vi "HYSTERISIS_TEMPERATURE CONTROL.vi"() -> ()   [LabVIEW 2010]
uses:
  <instrlib>/Keithley 24XX/Public/Data/Read (Multiple Points).vi
  <vilib>/Utility/file.llb/Write To Spreadsheet File (DBL).vi
  C/Program Files/National Instruments/LabVIEW 2016/instr.lib/Stanford Research 830/Stanford Research 830.lvlib
  C/Program Files/National Instruments/LabVIEW 2016/instr.lib/Keithley 2450/Keithley 2450.lvlib
  <instrlib>/Keithley 24XX/Keithley 24XX.lvlib
  <vilib>/Analysis/NI_AALBase.lvlib
  C/Program Files/National Instruments/LabVIEW 2016/instr.lib/Lake Shore Cryotronics 331/Lake Shore Cryotronics 331.lvlib
panel:
  out "Kelvin Reading 3":dbl min=0.0 max=1645.0 step=1e-05 format="%^.5e"
  in  "Input (0: A) 3":u16(ring) items=["A", "B"]
  out "TEMPERATURE SET":i32
  out "Loop 1\nHeater Output 2":dbl(slide) min=0.0 max=100.0 step=0.01 scale=0.0..100.0 scale format="%.1f"
  in  "Input (0: A) 2":u16(ring) items=["A", "B"]
  out "Kelvin Reading 2":dbl min=0.0 max=1645.0 step=1e-05 format="%^.5e"
  in  "TEMPERATURE STABLE TIME":i32=1000
  in  "TEMPERATURE POINT":i32
  in  "TEMPERATURE SPACE":i32
  in  "INITIAL temperature":i32
  in  "Loop (0: 1)":u16(ring) items=["1", "2"]
  in  "LAKESHORE":refnum<visa-resource-name>="GPIB0::12::INSTR"
  in  "Gain (P) (0.0)":dbl min=0.0 max=1000.0 step=0.1 format="%.1f"
  in  "Reset (I) (0.0)":dbl min=0.0 max=1000.0 step=0.1 format="%.1f"
  in  "Manual Output (0.000)":dbl min=0.0 max=100.0 step=0.001 format="%.3f"
  in  "Heater Range (0: Off)":u16(ring) items=["Off", "Low (0.5W)", "Med (5W)", "High (50W)"]
  in  "Rate (D) (0)":dbl min=0.0 max=200.0 step=1.0
  in  "Configure (False)":bool
  in  "Parameter2 (1: X)  2":u16(ring)=4 items=["X"=1, "Y"=2, "R"=3, "Theta"=4, "Channel 1"=5, "Channel 2"=6, "Aux In 1"=7, "Aux In 2"=8, "Aux In 3"=9, "Aux In 4"=10]
  out "PHASE":dbl=180.0
  out "LOCKIN2\n-THETA":cluster{dbl[], dbl[]}(graph)={[0.0, 0.0, 0.0, 0.0, 0.0, 0.0, 2.3842e-07, 0.0, 0.0, 0.0, 0.0, 0.0, 0.0, 0.0, 0.0, 0.0, 0.0, 0.0, 0.0, 0.0, 0.0, 0.0, 2.3842e-07, 2.3842e-07, 4.76841e-07, 2.3842e-07, 2.3842e-07, 0.0, 0.0, 0.0, 0.0, 0.0, 0.0, 0.0, 0.0, 0.0, 0.0, 2.3842e-07, 2.3842e-07, 2.3842e-07, 0.0, 2.3842e-07, 2.3842e-07, 0.0, 0.0, 0.0, 0.0, 0.0, 0.0, 0.0, 0.0, 0.0, 0.0, 0.0, 2.3842e-07, 2.3842e-07, 2.3842e-07, 2.3842e-07, 0.0, 0.0, 0.0, 0.0, 0.0, 0.0, 0.0, 0.0, 0.0, 0.0, 0.0, 0.0, 0.0, 0.0, 0.0, 0.0, 0.0, 0.0, 0.0, 0.0, 0.0, 0.0, 0.0, 0.0, 0.0, 0.0, 0.0, 0.0, 0.0, 0.0, 0.0, 0.0, 0.0, 0.0, 0.0, 0.0, 0.0, 0.0, 0.0, 0.0, 0.0, 0.0, 0.0, 0.0, 0.0, 0.0, 0.0, 2.3842e-07, 2.3842e-07, 2.3842e-07, 0.0, 0.0, 0.0, 0.0, 0.0, 0.0, 0.0, 0.0, 0.0, 0.0, 0.0, 2.3842e-07, 2.3842e-07, 2.3842e-07, 2.3842e-07, 2.3842e-07, 0.0, 2.3842e-07, 2.3842e-07, 2.3842e-07, 2.3842e-07, 0.0, 0.0, 0.0, 0.0, 0.0, 0.0, 0.0, 0.0, 0.0, 0.0, 0.0, 0.0, 0.0, 0.0, 0.0, 0.0, 0.0, 0.0, 0.0, 0.0, 0.0, 0.0, 4.76841e-07, 9.53682e-07, 1.66894e-06, 2.62262e-06, 4.29156e-06, 6.43733e-06, 9.77522e-06, 1.33515e-05, 1.59742e-05, 1.57357e-05, 7.86787e-06, 9.53682e-07, 0.0, 0.0, 2.3842e-07, 2.3842e-07, 2.3842e-07, 2.3842e-07, 0.0, 0.0, 0.0, 0.0, 0.0, 0.0, 0.0, 0.0, 0.0, 0.0, 2.3842e-07, 2.3842e-07, 2.3842e-07, 0.0, 0.0, 0.0, 0.0, 0.0, 0.0, 0.0, 0.0, 0.0, 0.0, 0.0, 0.0, 0.0, 0.0, 0.0, 2.3842e-07, 2.3842e-07, 2.3842e-07, 4.76841e-07, 2.3842e-07, 0.0, 0.0, 0.0, 0.0, 0.0, 0.0, 0.0, 0.0, 0.0, 0.0, 0.0, 0.0, 0.0, 0.0, 0.0, 0.0, 0.0, 0.0, 0.0, 0.0, 0.0, 0.0, 0.0, 0.0, 0.0, 0.0, 0.0, 0.0, 0.0, 0.0, 0.0, 0.0, 0.0, 0.0, 0.0, 0.0, 0.0, 0.0, 2.3842e-07, 0.0, 2.3842e-07, 2.3842e-07, 2.3842e-07, 2.3842e-07, 2.3842e-07, 0.0, 0.0, 0.0, 0.0, 0.0, 2.3842e-07, 2.3842e-07, 4.76841e-07, 4.76841e-07, 4.76841e-07, 2.3842e-07, 2.3842e-07, 0.0, 0.0, 0.0, 0.0, 0.0, 0.0, 0.0, 0.0, 2.3842e-07, 2.3842e-07, 2.3842e-07, 2.3842e-07, 2.3842e-07, 2.3842e-07, 2.3842e-07, 2.3842e-07, 2.3842e-07, 2.3842e-07, 2.3842e-07, 2.3842e-07, 2.3842e-07, 2.3842e-07, 2.3842e-07, 2.3842e-07, 0.0, 0.0, 0.0, 0.0, 0.0, 0.0, 2.3842e-07, 2.3842e-07, 2.3842e-07, 2.3842e-07, 2.3842e-07, 2.3842e-07, 2.3842e-07, 0.0], [180.0, 135.0, 90.0, 45.0, 45.0, 45.0, 0.0, 0.0, 0.0, 0.0, 0.0, 45.0, 45.0, 45.0, 45.0, 45.0, 45.0, 45.0, 45.0, 45.0, 90.0, 90.0, 116.562, 116.562, 108.432, 116.562, 116.562, 135.0, 135.0, 0.0, 0.0, 0.0, 45.0, 45.0, 45.0, 45.0, 45.0, 26.562, 26.562, 0.0, -45.0, -45.0, -63.438, -90.0, -45.0, -45.0, 0.0, 0.0, 0.0, 0.0, 0.0, 0.0, 90.0, 45.0, 26.562, 26.562, 26.562, 26.562, 45.0, 90.0, 90.0, 0.0, 0.0, -90.0, -90.0, -90.0, -90.0, 0.0, 0.0, 0.0, 0.0, 0.0, 0.0, 90.0, 90.0, 90.0, 90.0, 180.0, -135.0, -135.0, -135.0, 0.0, 0.0, 0.0, 0.0, -45.0, 0.0, 45.0, 45.0, 45.0, 45.0, 45.0, 45.0, 90.0, 0.0, 0.0, -90.0, -90.0, -90.0, -90.0, 0.0, 0.0, 45.0, 45.0, 45.0, 63.438, 63.438, 90.0, 45.0, 90.0, 90.0, 0.0, 0.0, -45.0, -45.0, -45.0, -45.0, -45.0, -45.0, -63.438, -63.438, -90.0, -90.0, -90.0, -63.438, -26.562, 0.0, 0.0, 26.562, 45.0, 45.0, 0.0, -45.0, -45.0, -90.0, 0.0, 45.0, 45.0, 0.0, 0.0, 0.0, 45.0, 45.0, 45.0, 45.0, 45.0, 90.0, 90.0, 135.0, 135.0, 90.0, 71.568, 59.034, 53.13, 49.764, 49.638, 49.086, 49.188, 49.554, 49.59, 49.968, 50.628, 56.31, 135.0, 135.0, 153.438, 180.0, 180.0, 180.0, 180.0, -135.0, -90.0, -90.0, -45.0, -45.0, -45.0, -45.0, -45.0, -45.0, 0.0, 26.562, 26.562, 45.0, 45.0, 0.0, 0.0, 0.0, 90.0, 90.0, 90.0, 45.0, 45.0, 45.0, 45.0, 0.0, -45.0, -45.0, -63.438, -63.438, -63.438, -45.0, -26.562, -45.0, -45.0, -45.0, -45.0, -90.0, -90.0, 0.0, 0.0, 0.0, 0.0, 0.0, 0.0, 0.0, -45.0, -45.0, -45.0, -90.0, 0.0, 90.0, 90.0, 90.0, 90.0, 45.0, 45.0, 45.0, 45.0, 45.0, 45.0, 0.0, 0.0, 0.0, 0.0, 0.0, -45.0, -45.0, -45.0, -90.0, -90.0, -63.438, -45.0, -26.562, 0.0, 0.0, -26.562, -26.562, -45.0, -45.0, -45.0, -45.0, -45.0, 0.0, 26.562, 18.432, 18.432, 18.432, 26.562, 26.562, 45.0, 45.0, 90.0, 90.0, 0.0, 0.0, -45.0, -45.0, -26.562, -26.562, -26.562, -26.562, 0.0, 0.0, 0.0, 0.0, 0.0, 0.0, 0.0, 0.0, 26.562, 26.562, 26.562, 0.0, 0.0, 0.0, 45.0, 45.0, 0.0, 0.0, 0.0, 0.0, 0.0, 26.562, 26.562, 0.0, 0.0, 0.0]}
  in  "Parameter (1: X) 2":u16(ring)=3 items=["X"=1, "Y"=2, "R"=3, "Theta"=4, "Channel 1"=5, "Channel 2"=6, "Aux In 1"=7, "Aux In 2"=8, "Aux In 3"=9, "Aux In 4"=10]
  out "R Measurement 2":dbl
  out "LOVK2-r":cluster{dbl[], dbl[]}(graph)={[0.0, 0.0, 0.0, 0.0, 0.0, 0.0, 2.3842e-07, 0.0, 0.0, 0.0, 0.0, 0.0, 0.0, 0.0, 0.0, 0.0, 0.0, 0.0, 0.0, 0.0, 0.0, 0.0, 2.3842e-07, 2.3842e-07, 4.76841e-07, 2.3842e-07, 2.3842e-07, 0.0, 0.0, 0.0, 0.0, 0.0, 0.0, 0.0, 0.0, 0.0, 0.0, 2.3842e-07, 2.3842e-07, 2.3842e-07, 0.0, 2.3842e-07, 2.3842e-07, 0.0, 0.0, 0.0, 0.0, 0.0, 0.0, 0.0, 0.0, 0.0, 0.0, 0.0, 2.3842e-07, 2.3842e-07, 2.3842e-07, 2.3842e-07, 0.0, 0.0, 0.0, 0.0, 0.0, 0.0, 0.0, 0.0, 0.0, 0.0, 0.0, 0.0, 0.0, 0.0, 0.0, 0.0, 0.0, 0.0, 0.0, 0.0, 0.0, 0.0, 0.0, 0.0, 0.0, 0.0, 0.0, 0.0, 0.0, 0.0, 0.0, 0.0, 0.0, 0.0, 0.0, 0.0, 0.0, 0.0, 0.0, 0.0, 0.0, 0.0, 0.0, 0.0, 0.0, 0.0, 0.0, 2.3842e-07, 2.3842e-07, 2.3842e-07, 0.0, 0.0, 0.0, 0.0, 0.0, 0.0, 0.0, 0.0, 0.0, 0.0, 0.0, 2.3842e-07, 2.3842e-07, 2.3842e-07, 2.3842e-07, 2.3842e-07, 0.0, 2.3842e-07, 2.3842e-07, 2.3842e-07, 2.3842e-07, 0.0, 0.0, 0.0, 0.0, 0.0, 0.0, 0.0, 0.0, 0.0, 0.0, 0.0, 0.0, 0.0, 0.0, 0.0, 0.0, 0.0, 0.0, 0.0, 0.0, 0.0, 0.0, 4.76841e-07, 9.53682e-07, 1.66894e-06, 2.62262e-06, 4.29156e-06, 6.43733e-06, 9.77522e-06, 1.33515e-05, 1.59742e-05, 1.57357e-05, 7.86787e-06, 9.53682e-07, 0.0, 0.0, 2.3842e-07, 2.3842e-07, 2.3842e-07, 2.3842e-07, 0.0, 0.0, 0.0, 0.0, 0.0, 0.0, 0.0, 0.0, 0.0, 0.0, 2.3842e-07, 2.3842e-07, 2.3842e-07, 0.0, 0.0, 0.0, 0.0, 0.0, 0.0, 0.0, 0.0, 0.0, 0.0, 0.0, 0.0, 0.0, 0.0, 0.0, 2.3842e-07, 2.3842e-07, 2.3842e-07, 4.76841e-07, 2.3842e-07, 0.0, 0.0, 0.0, 0.0, 0.0, 0.0, 0.0, 0.0, 0.0, 0.0, 0.0, 0.0, 0.0, 0.0, 0.0, 0.0, 0.0, 0.0, 0.0, 0.0, 0.0, 0.0, 0.0, 0.0, 0.0, 0.0, 0.0, 0.0, 0.0, 0.0, 0.0, 0.0, 0.0, 0.0, 0.0, 0.0, 0.0, 0.0, 2.3842e-07, 0.0, 2.3842e-07, 2.3842e-07, 2.3842e-07, 2.3842e-07, 2.3842e-07, 0.0, 0.0, 0.0, 0.0, 0.0, 2.3842e-07, 2.3842e-07, 4.76841e-07, 4.76841e-07, 4.76841e-07, 2.3842e-07, 2.3842e-07, 0.0, 0.0, 0.0, 0.0, 0.0, 0.0, 0.0, 0.0, 2.3842e-07, 2.3842e-07, 2.3842e-07, 2.3842e-07, 2.3842e-07, 2.3842e-07, 2.3842e-07, 2.3842e-07, 2.3842e-07, 2.3842e-07, 2.3842e-07, 2.3842e-07, 2.3842e-07, 2.3842e-07, 2.3842e-07, 2.3842e-07, 0.0, 0.0, 0.0, 0.0, 0.0, 0.0, 2.3842e-07, 2.3842e-07, 2.3842e-07, 2.3842e-07, 2.3842e-07, 2.3842e-07, 2.3842e-07, 0.0], [0.0, 0.0, 0.0, 0.0, 0.0, 0.0, 2.3842e-07, 0.0, 0.0, 0.0, 0.0, 0.0, 0.0, 0.0, 0.0, 0.0, 0.0, 0.0, 0.0, 0.0, 0.0, 0.0, 2.3842e-07, 2.3842e-07, 4.76841e-07, 2.3842e-07, 2.3842e-07, 0.0, 0.0, 0.0, 0.0, 0.0, 0.0, 0.0, 0.0, 0.0, 0.0, 2.3842e-07, 2.3842e-07, 2.3842e-07, 0.0, 2.3842e-07, 2.3842e-07, 0.0, 0.0, 0.0, 0.0, 0.0, 0.0, 0.0, 0.0, 0.0, 0.0, 0.0, 2.3842e-07, 2.3842e-07, 2.3842e-07, 2.3842e-07, 0.0, 0.0, 0.0, 0.0, 0.0, 0.0, 0.0, 0.0, 0.0, 0.0, 0.0, 0.0, 0.0, 0.0, 0.0, 0.0, 0.0, 0.0, 0.0, 0.0, 0.0, 0.0, 0.0, 0.0, 0.0, 0.0, 0.0, 0.0, 0.0, 0.0, 0.0, 0.0, 0.0, 0.0, 0.0, 0.0, 0.0, 0.0, 0.0, 0.0, 0.0, 0.0, 0.0, 0.0, 0.0, 0.0, 0.0, 2.3842e-07, 2.3842e-07, 2.3842e-07, 0.0, 0.0, 0.0, 0.0, 0.0, 0.0, 0.0, 0.0, 0.0, 0.0, 0.0, 2.3842e-07, 2.3842e-07, 2.3842e-07, 2.3842e-07, 2.3842e-07, 0.0, 2.3842e-07, 2.3842e-07, 2.3842e-07, 2.3842e-07, 0.0, 0.0, 0.0, 0.0, 0.0, 0.0, 0.0, 0.0, 0.0, 0.0, 0.0, 0.0, 0.0, 0.0, 0.0, 0.0, 0.0, 0.0, 0.0, 0.0, 0.0, 0.0, 4.76841e-07, 9.53682e-07, 1.66894e-06, 2.62262e-06, 4.29156e-06, 6.43733e-06, 9.77522e-06, 1.33515e-05, 1.59742e-05, 1.57357e-05, 7.86787e-06, 9.53682e-07, 0.0, 0.0, 2.3842e-07, 2.3842e-07, 2.3842e-07, 2.3842e-07, 0.0, 0.0, 0.0, 0.0, 0.0, 0.0, 0.0, 0.0, 0.0, 0.0, 2.3842e-07, 2.3842e-07, 2.3842e-07, 0.0, 0.0, 0.0, 0.0, 0.0, 0.0, 0.0, 0.0, 0.0, 0.0, 0.0, 0.0, 0.0, 0.0, 0.0, 2.3842e-07, 2.3842e-07, 2.3842e-07, 4.76841e-07, 2.3842e-07, 0.0, 0.0, 0.0, 0.0, 0.0, 0.0, 0.0, 0.0, 0.0, 0.0, 0.0, 0.0, 0.0, 0.0, 0.0, 0.0, 0.0, 0.0, 0.0, 0.0, 0.0, 0.0, 0.0, 0.0, 0.0, 0.0, 0.0, 0.0, 0.0, 0.0, 0.0, 0.0, 0.0, 0.0, 0.0, 0.0, 0.0, 0.0, 2.3842e-07, 0.0, 2.3842e-07, 2.3842e-07, 2.3842e-07, 2.3842e-07, 2.3842e-07, 0.0, 0.0, 0.0, 0.0, 0.0, 2.3842e-07, 2.3842e-07, 4.76841e-07, 4.76841e-07, 4.76841e-07, 2.3842e-07, 2.3842e-07, 0.0, 0.0, 0.0, 0.0, 0.0, 0.0, 0.0, 0.0, 2.3842e-07, 2.3842e-07, 2.3842e-07, 2.3842e-07, 2.3842e-07, 2.3842e-07, 2.3842e-07, 2.3842e-07, 2.3842e-07, 2.3842e-07, 2.3842e-07, 2.3842e-07, 2.3842e-07, 2.3842e-07, 2.3842e-07, 2.3842e-07, 0.0, 0.0, 0.0, 0.0, 0.0, 0.0, 2.3842e-07, 2.3842e-07, 2.3842e-07, 2.3842e-07, 2.3842e-07, 2.3842e-07, 2.3842e-07, 0.0]}
  in  "Clear Plot 2":bool
  in  "TRIGGER (1:EXTERNAL)":i32=1
  in  "REFERENCE(0:EXTERNAL)":i32
  in  "auto phase 2":bool=TRUE
  in  "manual phase 2":dbl
  in  "harm#2 2":dbl=1.0
  in  "Sine Output Amplitude (1 V) 3":dbl=0.05
  in  "Input Connection (0: Single-Ended Voltage)  2":u16(ring)=1 items=["Single-Ended Voltage", "Differential Voltage", "1 MOhm Current Gain", "100 MOhm Current Gain"]
  in  "frequency 2":dbl=50.0 format="%#_13g"
  in  "lockin-NL":refnum<visa-resource-name>="GPIB0::10::INSTR"
  out "XY Graph 2":cluster{dbl[], dbl[]}(graph)={[0.0, -0.5, -1.0, -1.5, -2.0, -2.5, -3.0, -3.5, -3.0, -2.5, -2.0, -1.5, -1.0, -0.5, 0.0, 0.5, 1.0, 1.5, 2.0, 2.5, 3.0, 3.5, 3.0, 2.5, 2.0, 1.5, 1.0, 0.5, 0.0, 1.64, 1.66, 1.68, 1.7, 1.72, 1.74, 1.76, 1.78, 1.8, 1.82, 1.8399999999999999, 1.8599999999999999, 1.88, 1.9, 1.92, 1.94, 1.96, 1.98, 2.0, 2.02, 2.04, 2.06, 2.08, 2.0999999999999996, 2.12, 2.1399999999999997, 2.16, 2.1799999999999997, 2.2, 2.2199999999999998, 2.24, 2.26, 2.2800000000000002, 2.3, 2.3200000000000003, 2.34, 2.36, 2.38, 2.4, 2.42, 2.44, 2.46, 2.48, 2.5, 2.52, 2.54, 2.56, 2.58, 2.6, 2.62, 2.64, 2.66, 2.6799999999999997, 2.7, 2.7199999999999998, 2.74, 2.76, 2.7800000000000002, 2.8, 2.82, 2.84, 2.86, 2.88, 2.9, 2.92, 2.94, 2.96, 2.98, 3.0, 3.02, 3.04, 3.06, 3.08, 3.1, 3.12, 3.14, 3.16, 3.18, 3.2, 3.2199999999999998, 3.24, 3.26, 3.28, 3.3, 3.32, 3.34, 3.36, 3.38, 3.4, 3.42, 3.44, 3.46, 3.48, 3.5, 3.48, 3.46, 3.44, 3.42, 3.4, 3.38, 3.36, 3.34, 3.3200000000000003, 3.3000000000000003, 3.2800000000000002, 3.2600000000000002, 3.24, 3.22, 3.2, 3.18, 3.16, 3.14, 3.12, 3.1, 3.08, 3.06, 3.04, 3.02, 3.0, 2.98, 2.96, 2.94, 2.92, 2.9, 2.88, 2.86, 2.84, 2.82, 2.8000000000000003, 2.7800000000000002, 2.7600000000000002, 2.74, 2.72, 2.7, 2.68, 2.66, 2.64, 2.62, 2.6, 2.58, 2.56, 2.54, 2.52, 2.5, 2.48, 2.46, 2.44, 2.42, 2.4, 2.38, 2.36, 2.34, 2.32, 2.3000000000000003, 2.2800000000000002, 2.2600000000000002, 2.24, 2.22, 2.2, 2.18, 2.16, 2.14, 2.12, 2.1, 2.08, 2.06, 2.04, 2.02, 2.0, 1.98, 1.96, 1.94, 1.92, 1.9000000000000001, 1.8800000000000001, 1.86, 1.84, 1.82, 1.8, 1.78, 1.76, 1.74, 1.72, 1.7, 1.68, 1.6600000000000001, 1.6400000000000001, 1.62, 1.6, 1.58, 1.56, 1.54, 1.52, 1.5, 1.48, 1.46, 1.44, 1.42, 1.4000000000000001, 1.3800000000000001, 1.36, 1.34, 1.32, 1.3, 1.28, 1.26, 1.24, 1.22, 1.2, 1.18, 1.16, 1.1400000000000001, 1.12, 1.1, 1.08, 1.06, 1.04, 1.02, 1.0, 0.98, 0.96, 0.9400000000000001, 0.92, 0.9, 0.88, 0.86, 0.84, 0.8200000000000001, 0.8, 0.78, 0.76, 0.74, 0.72, 0.7000000000000001, 0.68, 0.66, 0.64, 0.62, 0.6, 0.58, 0.56, 0.54, 0.52, 0.5, 0.48, 0.46, 0.44, 0.42, 0.4, 0.38, 0.36, 0.34, 0.32, 0.3, 0.28, 0.26, 0.24, 0.22, 0.2, 0.18, 0.16, 0.14, 0.12, 0.1, 0.08, 0.06, 0.04, 0.02, 0.0], [180.0, 180.0, 180.0, -135.0, -90.0, -45.0, -63.438, -45.0, 45.0, 71.568, 71.568, 71.568, 90.0, 135.0, 135.0, 135.0, 180.0, -90.0, -90.0, -135.0, 0.0, 0.0, 0.0, -45.0, -45.0, -90.0, -90.0, 0.0, 90.0, -90.0, -45.0, 0.0, 0.0, -18.432, -18.432, -14.034, 0.0, 26.562, 26.562, 45.0, 33.69, 33.69, 18.432, 18.432, 18.432, 18.432, 0.0, 0.0, 0.0, 0.0, 90.0, 90.0, 90.0, 63.438, 90.0, 63.438, 90.0, 90.0, 180.0, -135.0, -90.0, -90.0, -45.0, -63.438, -90.0, -90.0, -90.0, -90.0, -90.0, -135.0, -116.562, -116.562, -116.562, -135.0, -116.562, -135.0, -135.0, 180.0, 135.0, 45.0, 63.438, 71.568, 63.438, 45.0, 0.0, -45.0, -45.0, -56.31, -45.0, -63.438, -63.438, -45.0, -90.0, -90.0, -90.0, -90.0, -90.0, -135.0, -153.438, -153.438, -135.0, -45.0, -45.0, -45.0, 0.0, 45.0, 45.0, 45.0, 45.0, 0.0, -90.0, -90.0, -90.0, -90.0, -63.438, -63.438, -63.438, -26.562, -18.432, -26.562, -26.562, -26.562, 0.0, 0.0, -18.432, -26.562, -63.438, -63.438, -63.438, -45.0, -45.0, -45.0, -45.0, -45.0, -45.0, -45.0, 0.0, 0.0, 45.0, 0.0, -18.432, -18.432, -33.69, -18.432, 0.0, 45.0, 45.0, 63.438, 63.438, 45.0, 26.562, 26.562, 26.562, 45.0, 26.562, 26.562, 18.432, 26.562, 45.0, 45.0, 45.0, 45.0, 45.0, 45.0, 45.0, 45.0, 63.438, 90.0, 90.0, 90.0, 90.0, 45.0, 90.0, 180.0, -135.0, -135.0, -90.0, -90.0, -90.0, -63.438, -45.0, -45.0, 0.0, 45.0, 45.0, -45.0, -45.0, -90.0, -63.438, -63.438, -45.0, -33.69, -33.69, -56.31, -71.568, -71.568, -71.568, -63.438, -71.568, -90.0, -45.0, 0.0, 45.0, 45.0, 63.438, 63.438, 71.568, 63.438, 63.438, 45.0, 90.0, 135.0, 180.0, 180.0, 153.438, 161.568, 180.0, 180.0, 180.0, 180.0, -90.0, -90.0, 0.0, 90.0, 90.0, 90.0, 0.0, -45.0, -45.0, -63.438, -63.438, -63.438, -71.568, -63.438, -63.438, -45.0, -45.0, -63.438, -45.0, -45.0, 0.0, 0.0, 45.0, 0.0, 0.0, 0.0, 90.0, 90.0, 90.0, 0.0, 0.0, 0.0, 0.0, 0.0, 0.0, 0.0, -26.562, -45.0, -45.0, -90.0, -90.0, 0.0, 45.0, 45.0, 63.438, 63.438, 63.438, 45.0, 63.438, 63.438, 63.438, 45.0, 0.0, -90.0, -90.0, -116.562, -135.0, 180.0, 135.0, 90.0, 45.0, 45.0, 0.0, -45.0, -63.438, -45.0, -71.568, -71.568, -63.438, -90.0, 0.0, 90.0, 63.438, 45.0, 26.562, 26.562, 0.0]}
  out "para2 Measurement":dbl=180.0
  in  "Parameter2 (1: X)":u16(ring)=4 items=["X"=1, "Y"=2, "R"=3, "Theta"=4, "Channel 1"=5, "Channel 2"=6, "Aux In 1"=7, "Aux In 2"=8, "Aux In 3"=9, "Aux In 4"=10]
  in  "auto phase":bool
  in  "manual phase":dbl
  in  "harm#2":dbl=2.0
  out "top gate leaking":dbl=-5.0360913356195525e-11
  out "top gate voltage":dbl=-0.0 format="%#_13g"
  in  "Compliance  Level (1uA)":dbl=2e-08
  in  "Source Mode  (0: Voltage)":u16(ring) items=["Voltage", "Current"]
  in  "top gate thickness":dbl=1.0
  in  "bottom gate thickness":dbl=1.0
  in  "pure field (T)/pure doping (F)":bool=TRUE
  in  "Serial Configuration":T1={"Baud Rate"=9600, "Parity"=0, "Data Bits"=8, "Stop Bits"=10, "Flow Control"=0} {"Flow Control" items=["None", "XON/XOFF", "RTS/CTS", "XON/XOFF & RTS/CTS", "DTR/DSR", "XON/XOFF & DTR/DSR"]; "Stop Bits" items=["1.0"=10, "1.5"=15, "2.0"=20]; "Data Bits" items=["7"=7, "8"=8]; "Parity" items=["None", "Odd", "Even", "Mark", "Space"]; "Baud Rate" items=["300"=300, "600"=600, "1200"=1200, "2400"=2400, "4800"=4800, "9600"=9600, "19200"=19200]}
  in  "top gate address":refnum<visa-resource-name>="GPIB0::25::INSTR"
  out "loop run":i32=1
  in  "loop #":i32=1
  in  "Save data or not":bool
  in  "path (folder + filename)":string="D:\\Kedar\\MoS2\\jw7_DJ_bulk_111213\\VvsHtr\\VvsHtr_300K"
  in  "Clear Plot":bool
  out "XY Graph":cluster{dbl[], dbl[]}(graph)={[0.0, -0.5, -1.0, -1.5, -2.0, -2.5, -3.0, -3.5, -3.0, -2.5, -2.0, -1.5, -1.0, -0.5, 0.0, 0.5, 1.0, 1.5, 2.0, 2.5, 3.0, 3.5, 3.0, 2.5, 2.0, 1.5, 1.0, 0.5, 0.0, 1.64, 1.66, 1.68, 1.7, 1.72, 1.74, 1.76, 1.78, 1.8, 1.82, 1.8399999999999999, 1.8599999999999999, 1.88, 1.9, 1.92, 1.94, 1.96, 1.98, 2.0, 2.02, 2.04, 2.06, 2.08, 2.0999999999999996, 2.12, 2.1399999999999997, 2.16, 2.1799999999999997, 2.2, 2.2199999999999998, 2.24, 2.26, 2.2800000000000002, 2.3, 2.3200000000000003, 2.34, 2.36, 2.38, 2.4, 2.42, 2.44, 2.46, 2.48, 2.5, 2.52, 2.54, 2.56, 2.58, 2.6, 2.62, 2.64, 2.66, 2.6799999999999997, 2.7, 2.7199999999999998, 2.74, 2.76, 2.7800000000000002, 2.8, 2.82, 2.84, 2.86, 2.88, 2.9, 2.92, 2.94, 2.96, 2.98, 3.0, 3.02, 3.04, 3.06, 3.08, 3.1, 3.12, 3.14, 3.16, 3.18, 3.2, 3.2199999999999998, 3.24, 3.26, 3.28, 3.3, 3.32, 3.34, 3.36, 3.38, 3.4, 3.42, 3.44, 3.46, 3.48, 3.5, 3.48, 3.46, 3.44, 3.42, 3.4, 3.38, 3.36, 3.34, 3.3200000000000003, 3.3000000000000003, 3.2800000000000002, 3.2600000000000002, 3.24, 3.22, 3.2, 3.18, 3.16, 3.14, 3.12, 3.1, 3.08, 3.06, 3.04, 3.02, 3.0, 2.98, 2.96, 2.94, 2.92, 2.9, 2.88, 2.86, 2.84, 2.82, 2.8000000000000003, 2.7800000000000002, 2.7600000000000002, 2.74, 2.72, 2.7, 2.68, 2.66, 2.64, 2.62, 2.6, 2.58, 2.56, 2.54, 2.52, 2.5, 2.48, 2.46, 2.44, 2.42, 2.4, 2.38, 2.36, 2.34, 2.32, 2.3000000000000003, 2.2800000000000002, 2.2600000000000002, 2.24, 2.22, 2.2, 2.18, 2.16, 2.14, 2.12, 2.1, 2.08, 2.06, 2.04, 2.02, 2.0, 1.98, 1.96, 1.94, 1.92, 1.9000000000000001, 1.8800000000000001, 1.86, 1.84, 1.82, 1.8, 1.78, 1.76, 1.74, 1.72, 1.7, 1.68, 1.6600000000000001, 1.6400000000000001, 1.62, 1.6, 1.58, 1.56, 1.54, 1.52, 1.5, 1.48, 1.46, 1.44, 1.42, 1.4000000000000001, 1.3800000000000001, 1.36, 1.34, 1.32, 1.3, 1.28, 1.26, 1.24, 1.22, 1.2, 1.18, 1.16, 1.1400000000000001, 1.12, 1.1, 1.08, 1.06, 1.04, 1.02, 1.0, 0.98, 0.96, 0.9400000000000001, 0.92, 0.9, 0.88, 0.86, 0.84, 0.8200000000000001, 0.8, 0.78, 0.76, 0.74, 0.72, 0.7000000000000001, 0.68, 0.66, 0.64, 0.62, 0.6, 0.58, 0.56, 0.54, 0.52, 0.5, 0.48, 0.46, 0.44, 0.42, 0.4, 0.38, 0.36, 0.34, 0.32, 0.3, 0.28, 0.26, 0.24, 0.22, 0.2, 0.18, 0.16, 0.14, 0.12, 0.1, 0.08, 0.06, 0.04, 0.02, 0.0], [0.0, 0.0, 0.0, 0.0, 0.0, 0.0, 1.1921e-07, 0.0, 0.0, 1.1921e-07, 1.1921e-07, 1.1921e-07, 1.1921e-07, 0.0, 0.0, 0.0, 0.0, 0.0, 0.0, 0.0, 0.0, 0.0, 0.0, 0.0, 0.0, 0.0, 0.0, 0.0, 0.0, 0.0, 0.0, 0.0, 0.0, 1.1921e-07, 1.1921e-07, 2.3842e-07, 1.1921e-07, 1.1921e-07, 1.1921e-07, 1.1921e-07, 2.3842e-07, 2.3842e-07, 1.1921e-07, 1.1921e-07, 1.1921e-07, 1.1921e-07, 1.1921e-07, 1.1921e-07, 0.0, 0.0, 0.0, 0.0, 0.0, 1.1921e-07, 1.1921e-07, 1.1921e-07, 0.0, 0.0, 0.0, 0.0, 0.0, 0.0, 1.1921e-07, 1.1921e-07, 1.1921e-07, 1.1921e-07, 0.0, 0.0, 0.0, 0.0, 1.1921e-07, 1.1921e-07, 1.1921e-07, 1.1921e-07, 1.1921e-07, 0.0, 0.0, 0.0, 0.0, 0.0, 1.1921e-07, 1.1921e-07, 1.1921e-07, 0.0, 0.0, 0.0, 1.1921e-07, 1.1921e-07, 1.1921e-07, 1.1921e-07, 1.1921e-07, 0.0, 0.0, 0.0, 0.0, 0.0, 0.0, 0.0, 1.1921e-07, 1.1921e-07, 0.0, 0.0, 0.0, 0.0, 1.1921e-07, 0.0, 0.0, 0.0, 0.0, 0.0, 0.0, 0.0, 0.0, 1.1921e-07, 1.1921e-07, 1.1921e-07, 1.1921e-07, 1.1921e-07, 1.1921e-07, 1.1921e-07, 1.1921e-07, 1.1921e-07, 1.1921e-07, 1.1921e-07, 1.1921e-07, 1.1921e-07, 1.1921e-07, 1.1921e-07, 1.1921e-07, 0.0, 0.0, 0.0, 0.0, 0.0, 0.0, 0.0, 0.0, 0.0, 0.0, 1.1921e-07, 1.1921e-07, 1.1921e-07, 2.3842e-07, 1.1921e-07, 0.0, 0.0, 1.1921e-07, 1.1921e-07, 1.1921e-07, 0.0, 1.1921e-07, 1.1921e-07, 1.1921e-07, 0.0, 1.1921e-07, 1.1921e-07, 1.1921e-07, 1.1921e-07, 0.0, 0.0, 0.0, 0.0, 0.0, 0.0, 0.0, 0.0, 1.1921e-07, 1.1921e-07, 0.0, 0.0, 0.0, 0.0, 0.0, 0.0, 0.0, 0.0, 1.1921e-07, 1.1921e-07, 1.1921e-07, 1.1921e-07, 0.0, 0.0, 0.0, 0.0, 0.0, 0.0, 0.0, 1.1921e-07, 1.1921e-07, 1.1921e-07, 1.1921e-07, 2.3842e-07, 2.3842e-07, 2.3842e-07, 1.1921e-07, 1.1921e-07, 1.1921e-07, 1.1921e-07, 1.1921e-07, 1.1921e-07, 0.0, 0.0, 0.0, 0.0, 1.1921e-07, 1.1921e-07, 1.1921e-07, 1.1921e-07, 1.1921e-07, 0.0, 0.0, 0.0, 0.0, 1.1921e-07, 1.1921e-07, 1.1921e-07, 1.1921e-07, 1.1921e-07, 0.0, 0.0, 0.0, 0.0, 0.0, 0.0, 0.0, 0.0, 0.0, 0.0, 0.0, 1.1921e-07, 1.1921e-07, 1.1921e-07, 1.1921e-07, 1.1921e-07, 1.1921e-07, 0.0, 0.0, 1.1921e-07, 0.0, 0.0, 0.0, 0.0, 0.0, 0.0, 0.0, 0.0, 0.0, 0.0, 0.0, 0.0, 0.0, 0.0, 1.1921e-07, 1.1921e-07, 1.1921e-07, 1.1921e-07, 1.1921e-07, 0.0, 0.0, 0.0, 0.0, 0.0, 0.0, 0.0, 1.1921e-07, 1.1921e-07, 0.0, 0.0, 1.1921e-07, 1.1921e-07, 1.1921e-07, 0.0, 0.0, 1.1921e-07, 1.1921e-07, 1.1921e-07, 0.0, 0.0, 0.0, 1.1921e-07, 0.0, 0.0, 0.0, 0.0, 1.1921e-07, 1.1921e-07, 1.1921e-07, 1.1921e-07, 1.1921e-07, 0.0, 0.0, 0.0, 1.1921e-07, 1.1921e-07, 1.1921e-07, 1.1921e-07, 1.1921e-07]}
  out "para1 Measurement":dbl
  in  "Parameter (1: X)":u16(ring)=3 items=["X"=1, "Y"=2, "R"=3, "Theta"=4, "Channel 1"=5, "Channel 2"=6, "Aux In 1"=7, "Aux In 2"=8, "Aux In 3"=9, "Aux In 4"=10]
  out "gate voltage":dbl format="%#_13g"
  out "gate leaking":string="1.034294E-10\n"
  in  "GATE STEP(mv)":i32=500
  in  "GATE Low Value (default 0)":dbl
  in  "GATE High Value":dbl=3.5
  in  "Function (0: Volts) 2":u16(ring) items=["Volts", "Current", "Resistance"]
  in  "Source Compaliance":dbl=1e-08
  in  "back gate address":refnum<visa-resource-name>="GPIB0::18::INSTR"
  in  "SD stabilization(S) 2":dbl=0.1 format="%#_13g"
  in  "Sine Output Amplitude (1 V) 2":dbl=0.2
  in  "LOCKIN-WAIT":dbl=0.1 format="%#_13g"
  in  "frequency":dbl=40.0 format="%#_13g"
  in  "Input Connection (0: Single-Ended Voltage)":u16(ring)=1 items=["Single-Ended Voltage", "Differential Voltage", "1 MOhm Current Gain", "100 MOhm Current Gain"]
  in  "LOCKIN address":refnum<visa-resource-name>="GPIB0::8::INSTR"
  # "Lock-in"
  # "top Gate Setting"
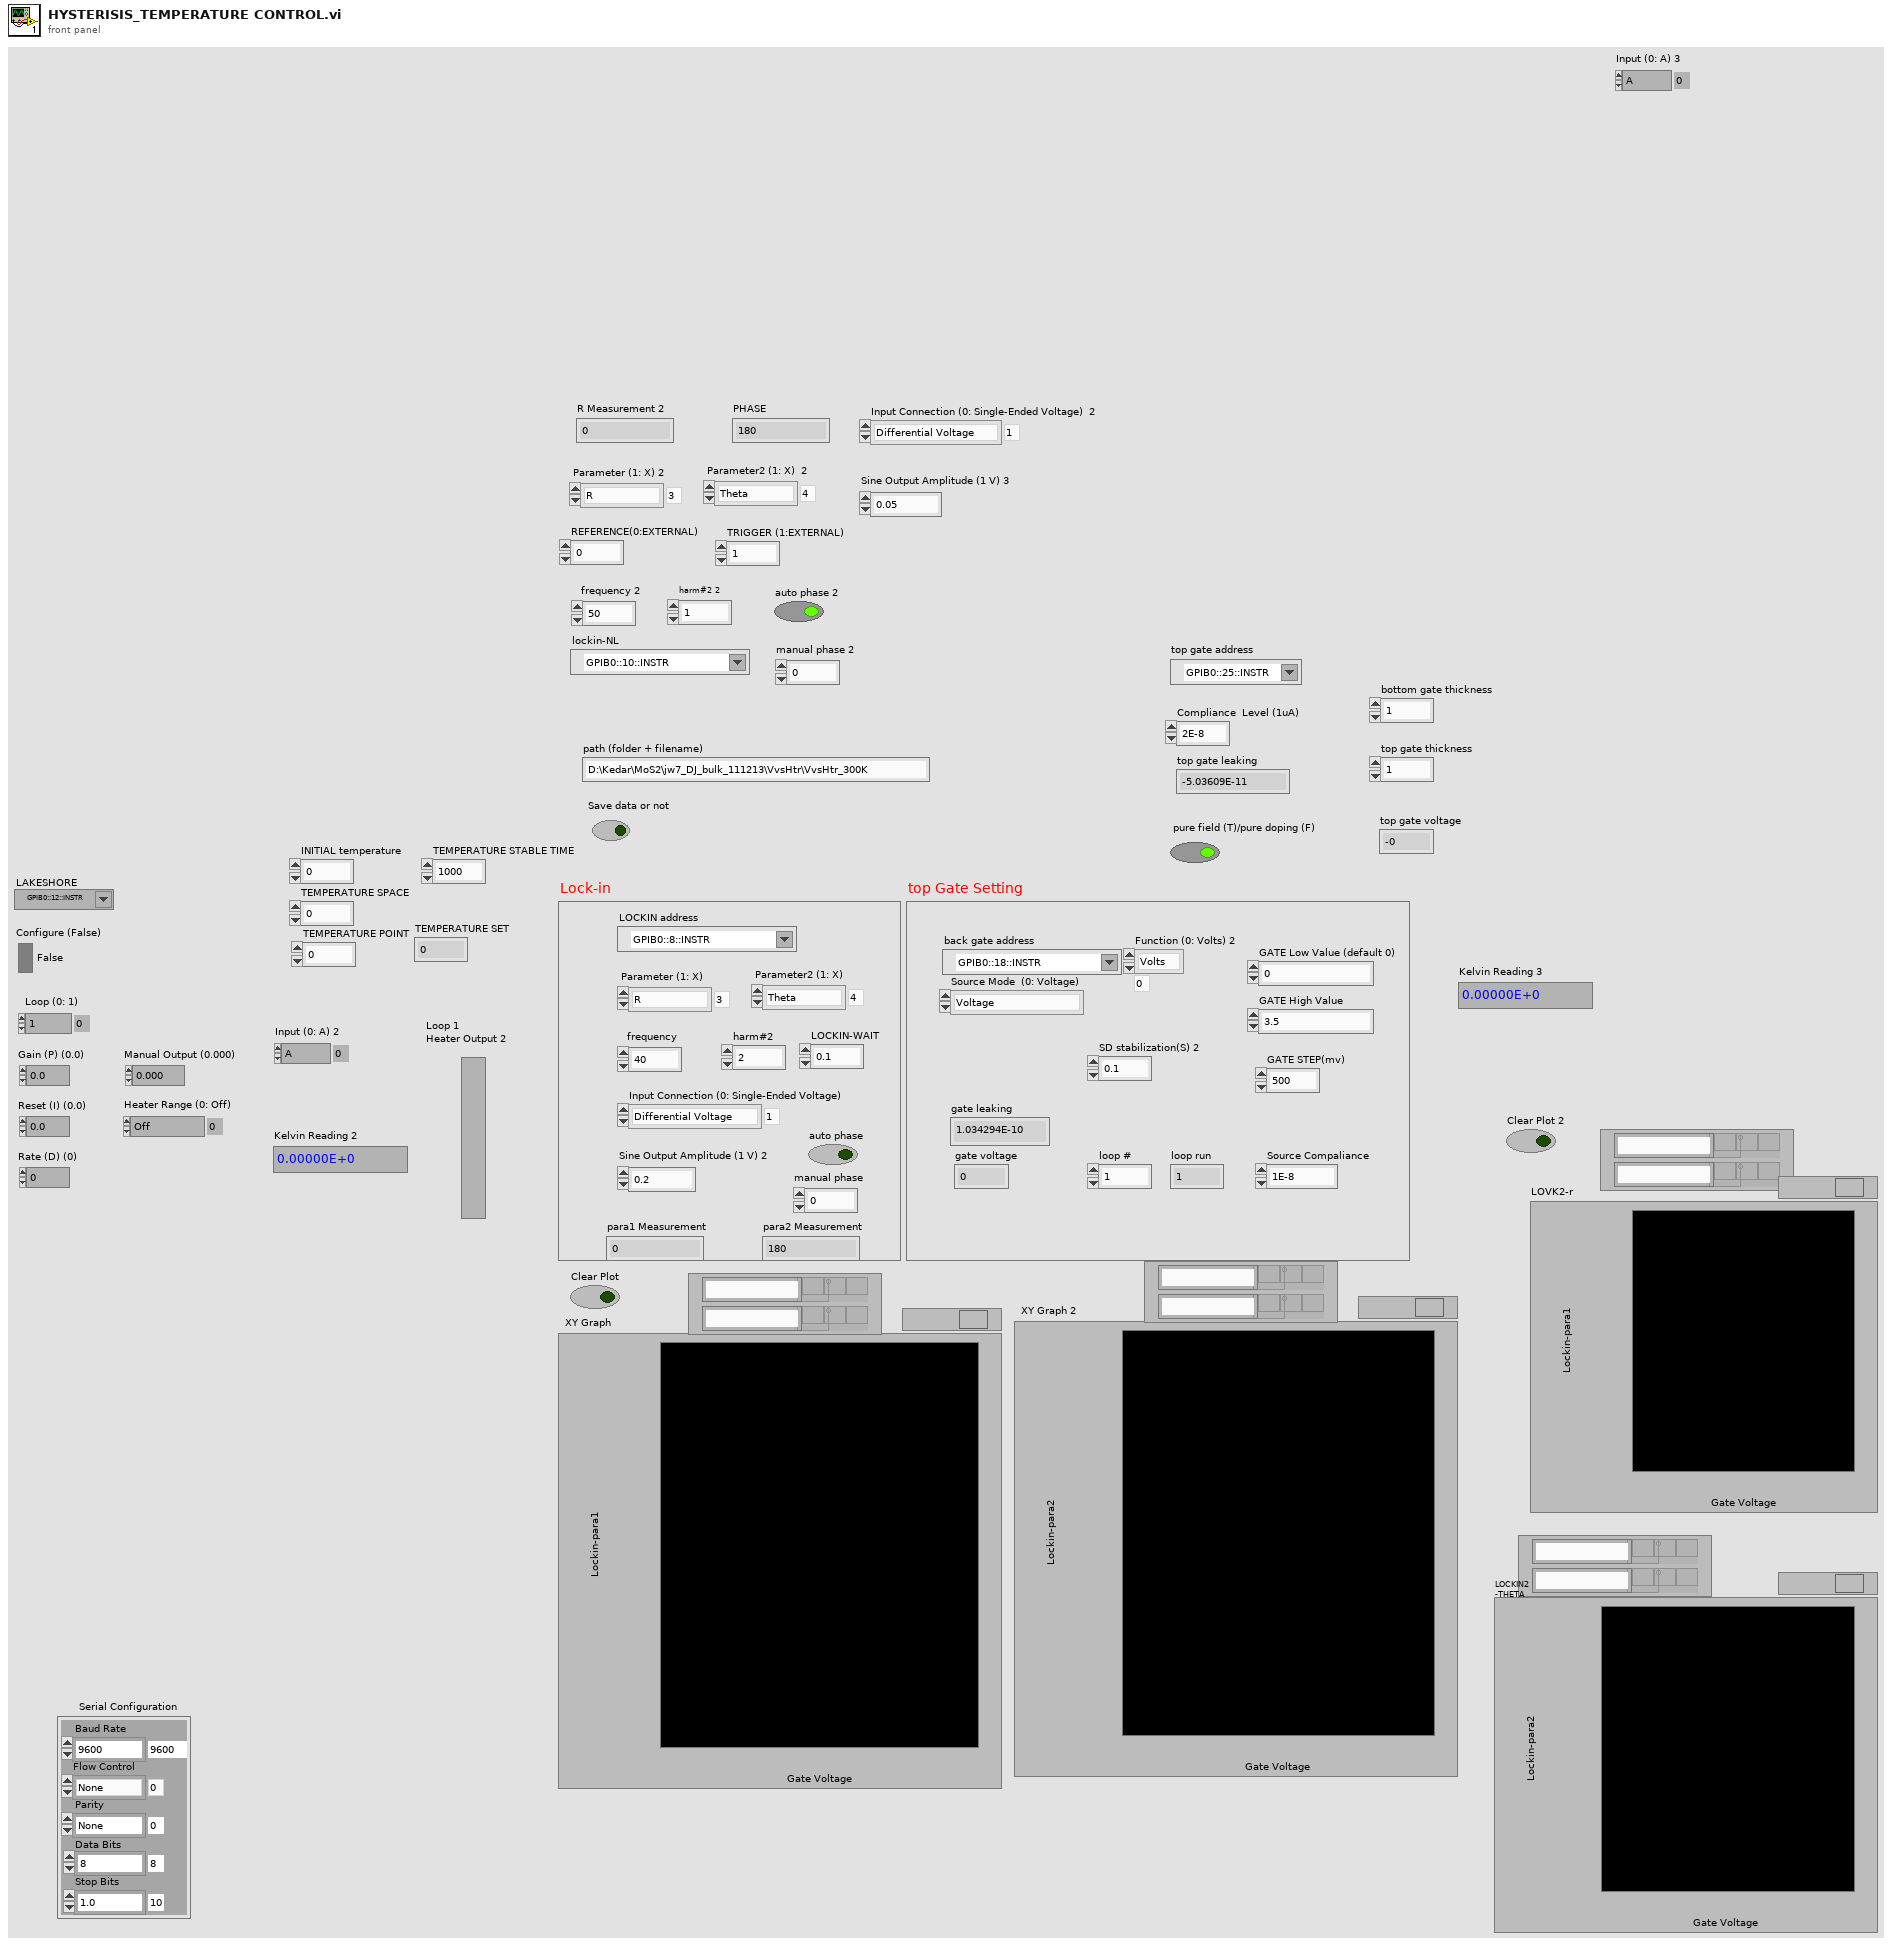
[diagram p1: front panel]
types:
  T1 = cluster{"Baud Rate":u32, "Parity":u16, "Data Bits":u16, "Stop Bits":u16, "Flow Control":u16}
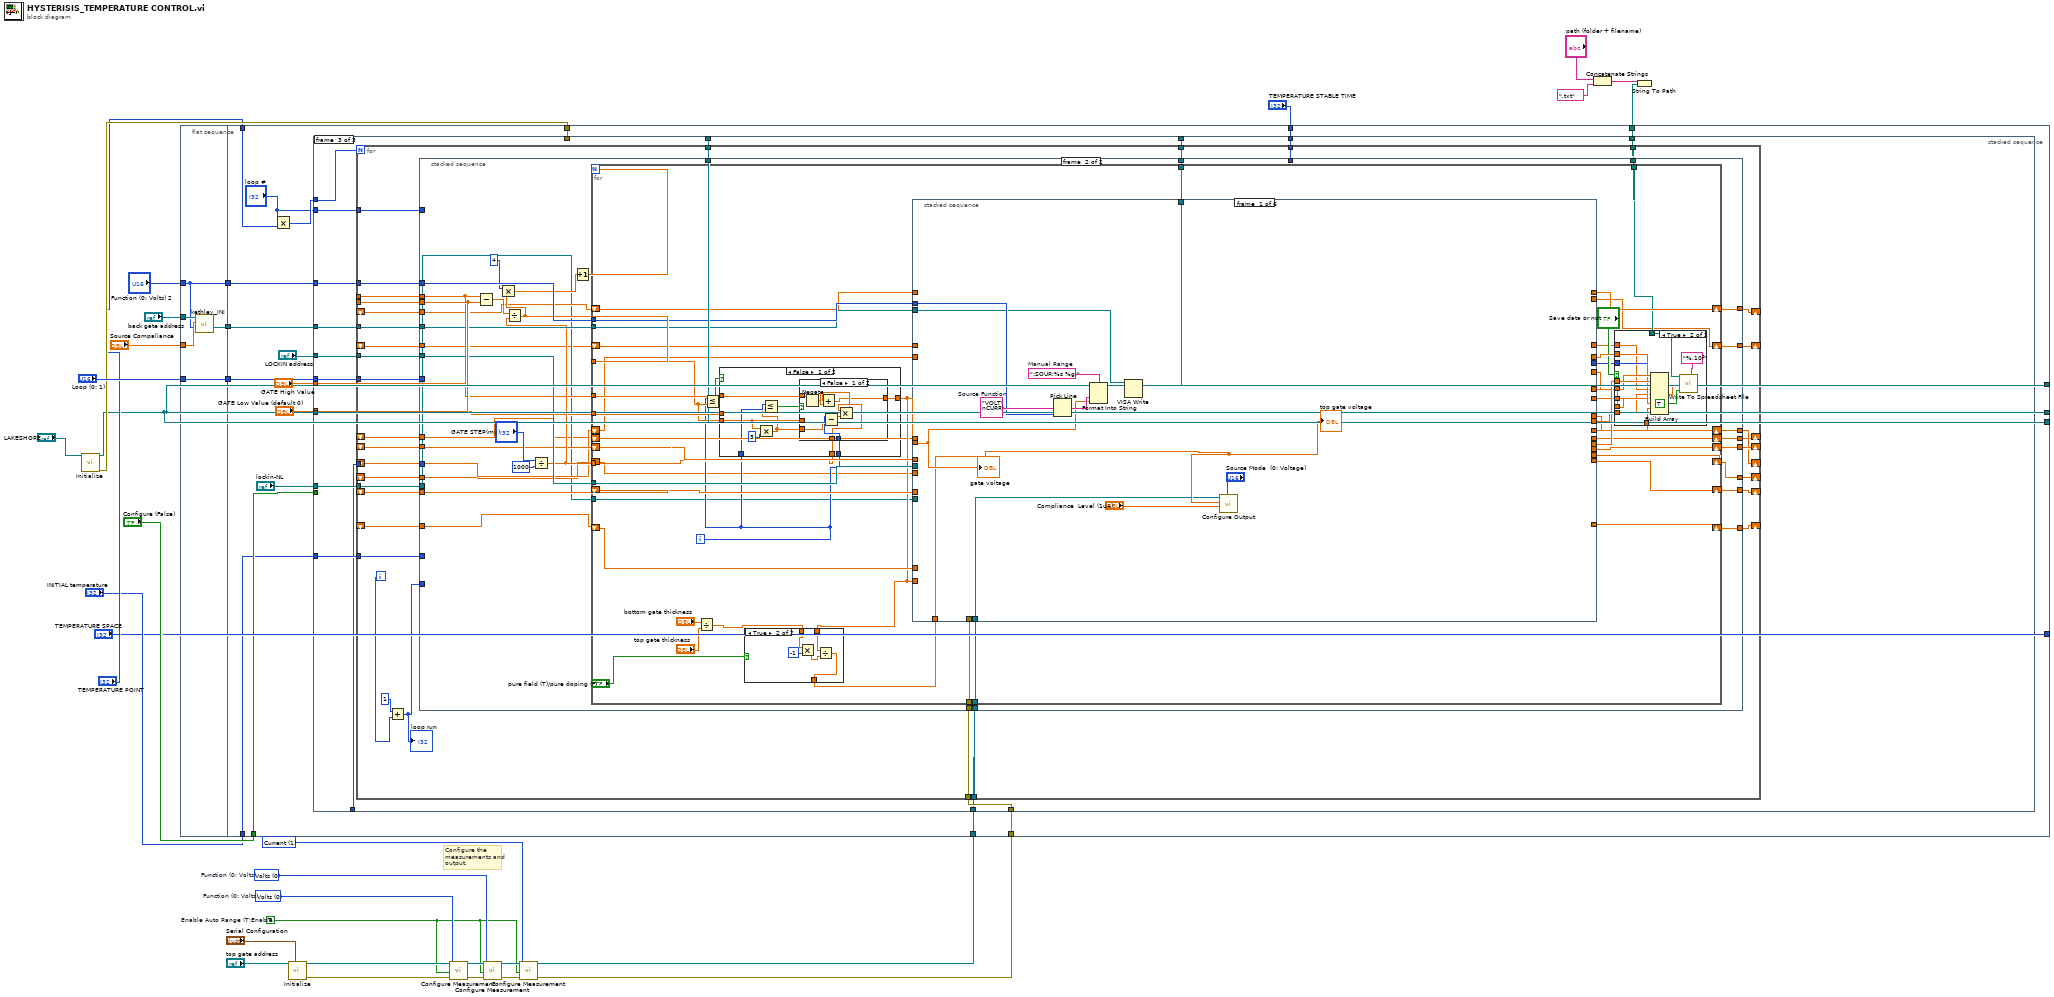
[diagram p0: block diagram]
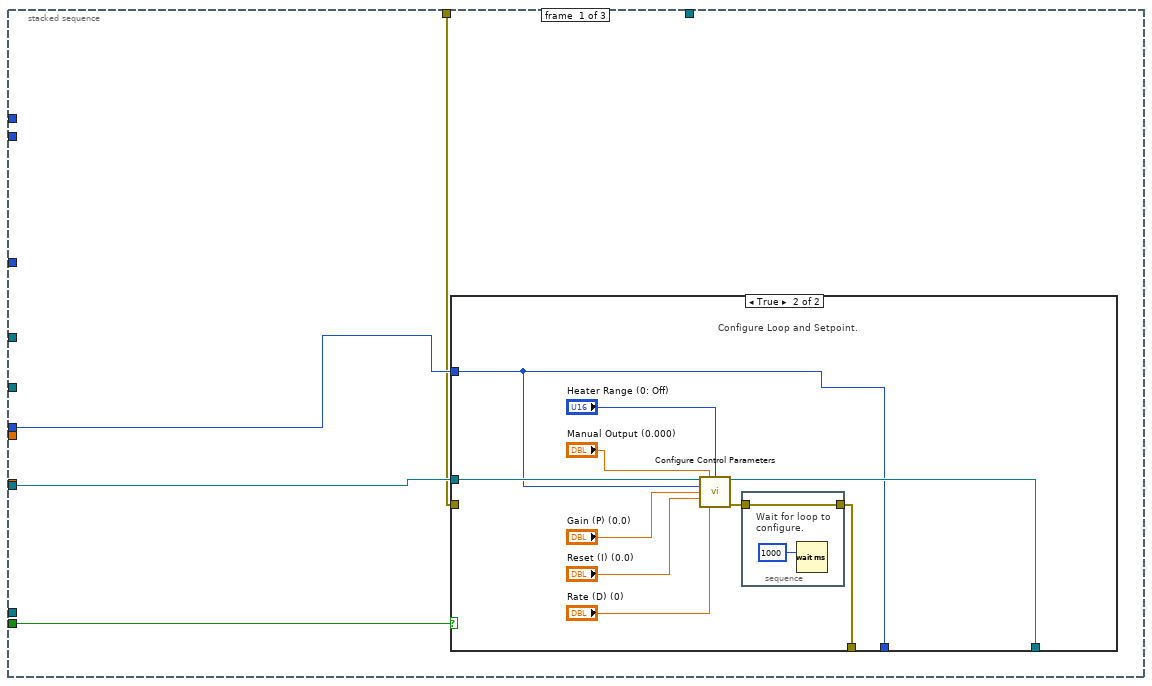
[diagram p2: hidden frame]
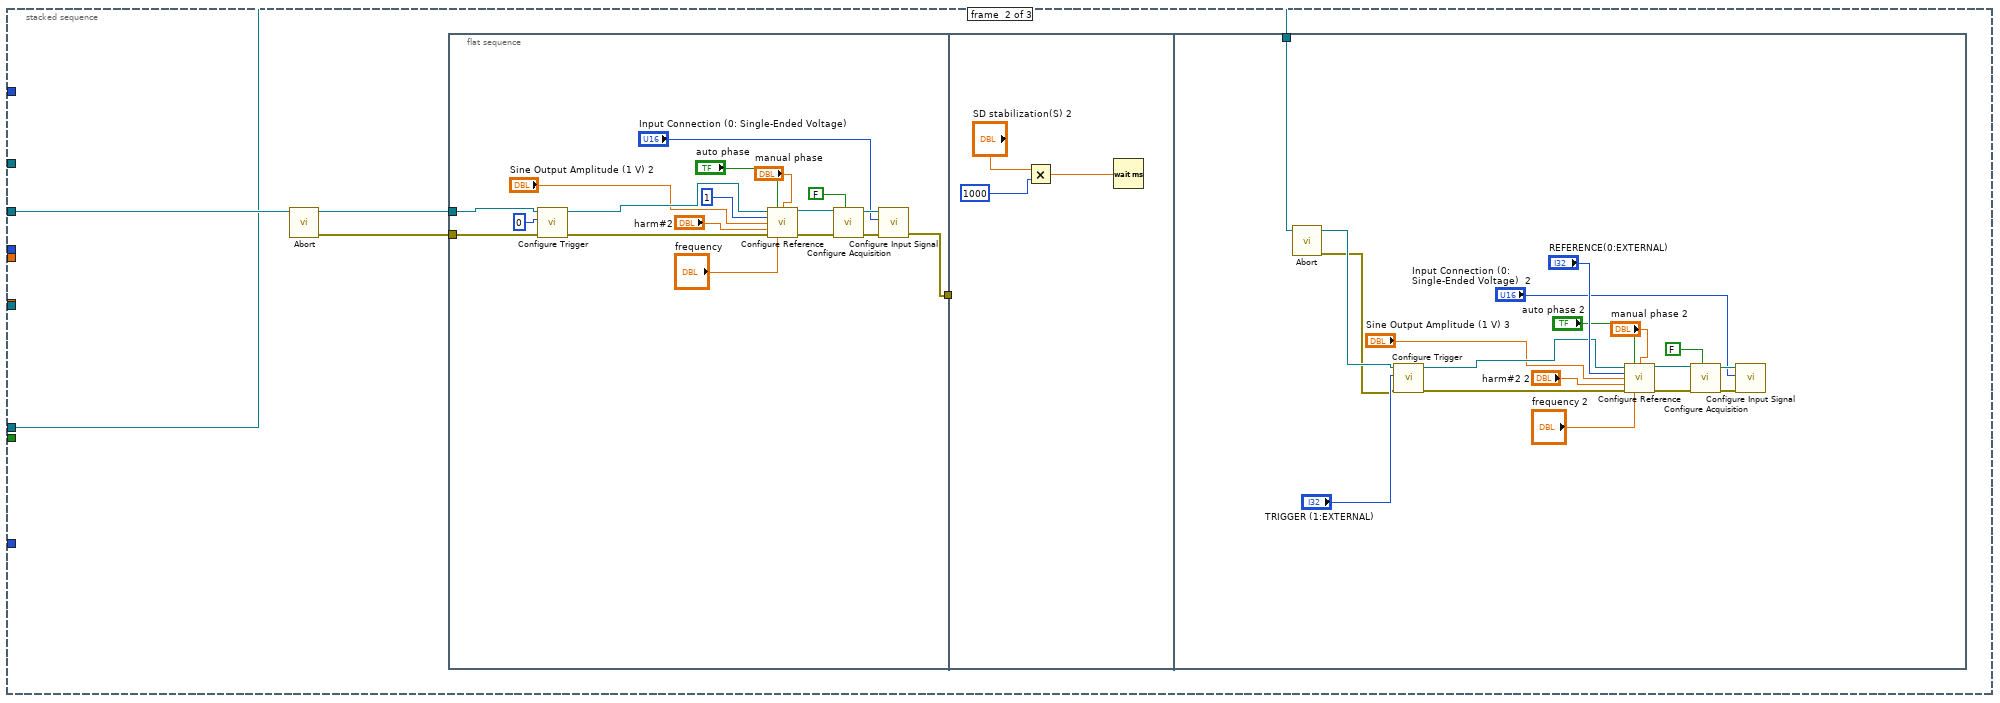
[diagram p4: hidden frame]
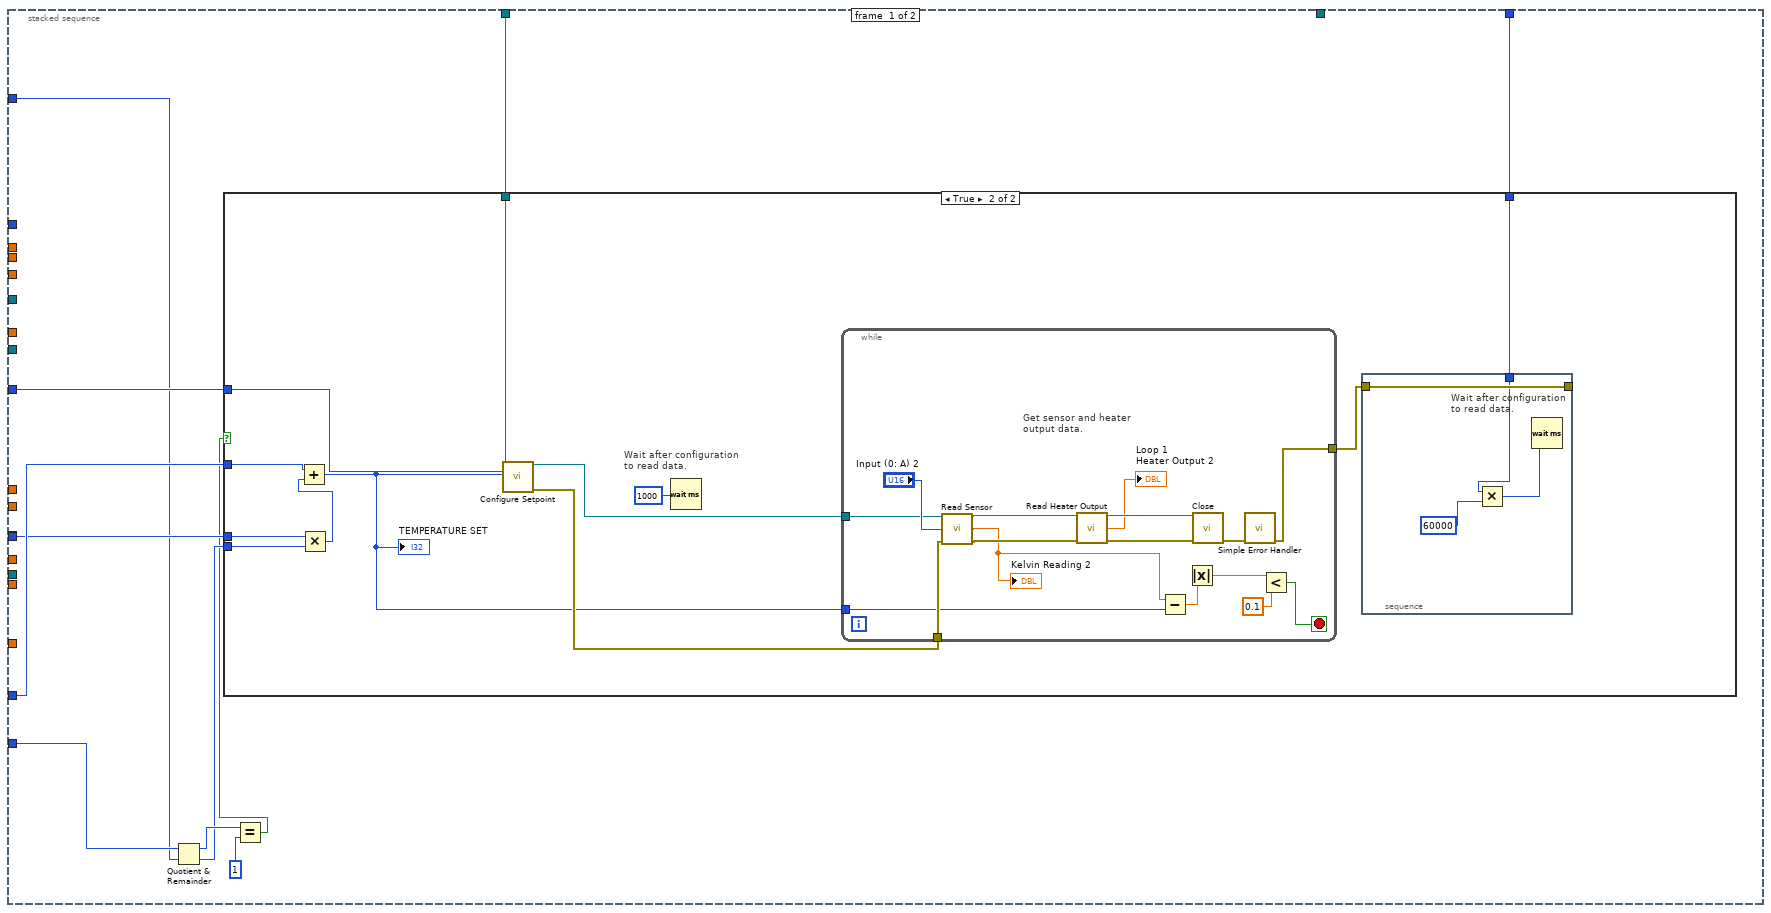
[diagram p5: hidden frame]
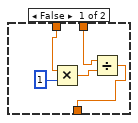
[diagram p7: hidden frame]
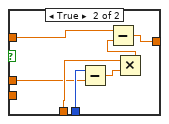
[diagram p9: hidden frame]
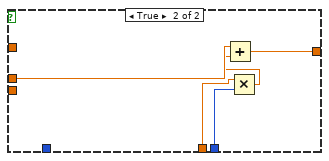
[diagram p10: hidden frame]
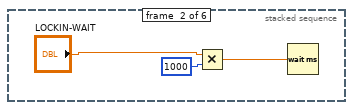
[diagram p11: hidden frame]
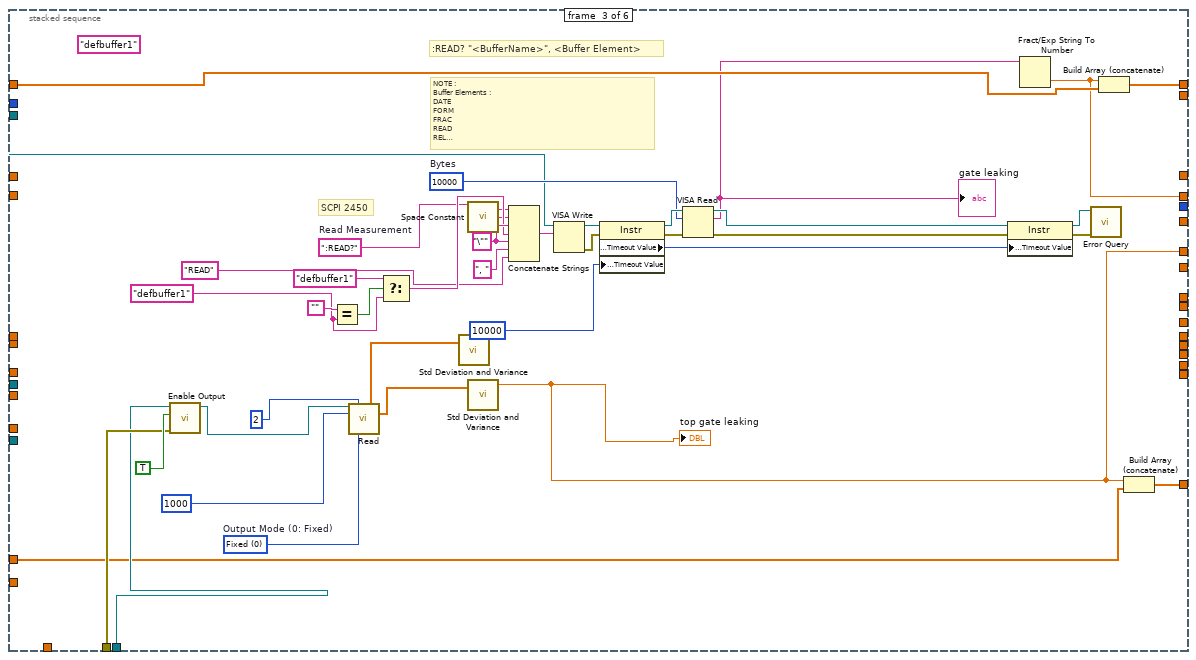
[diagram p12: hidden frame]
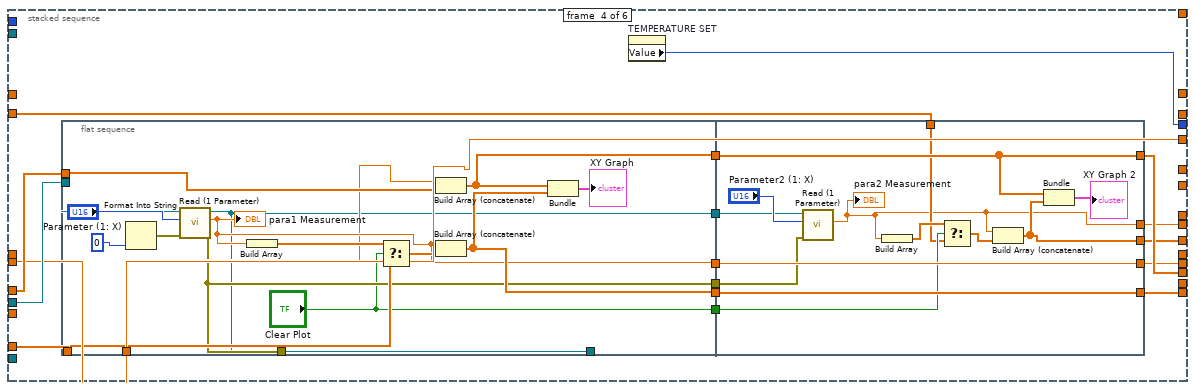
[diagram p13: hidden frame]
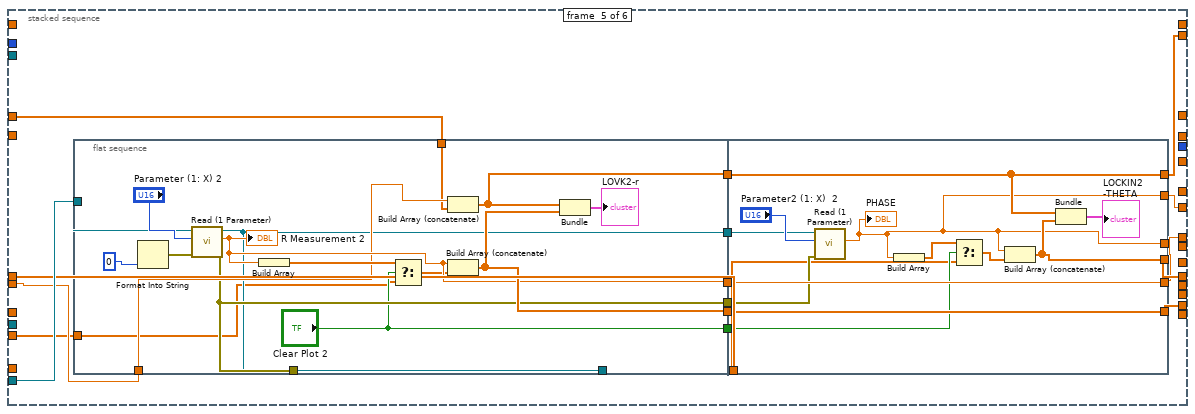
[diagram p14: hidden frame]
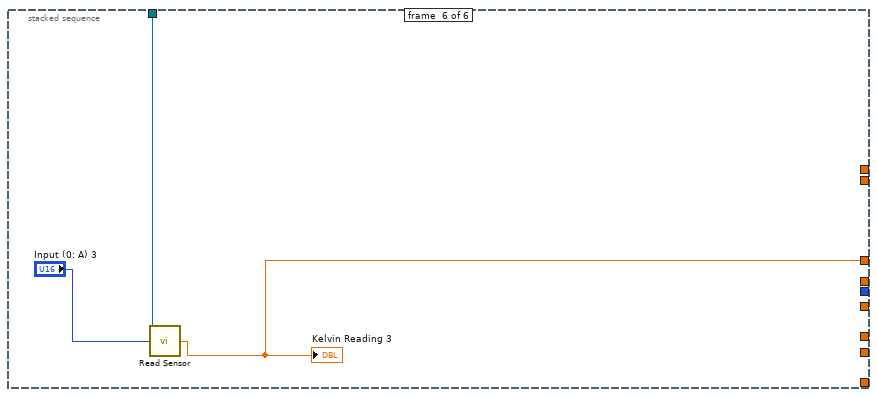
[diagram p15: hidden frame]
diagram:
  w13 = u16 1 items=["Volts", "Current", "Resistance"] ("Function (0: Volts)")
  w14 = TRUE  # Enable Auto Range (T:Enable)
  w17 = u16 0 items=["Volts", "Current", "Resistance"]  # Function (0: Volts)
  w18 = u16 0 items=["Volts", "Current", "Resistance"]  # Function (0: Volts)
  # "Configure the measurements and output."
  n1 = call <instrlib>:"Initialize.vi"("VISA resource name"="LAKESHORE") -> ("VISA resource name out"=w1:refnum<visa-resource-name>, "error out"=w7:errorcluster)  [unwired: 13 in]
  n2 = flat-sequence {
    tunnel: "back gate address" -> [w38]
    tunnel: "Source Compaliance" -> [w37]
    tunnel: "Function (0: Volts) 2" -> [w35]
    tunnel: [w36] -> w30
    tunnel: [w35] -> w29
    tunnel: [w34] -> w9
    tunnel: "Loop (0: 1)" -> [w34]
    tunnel: w30 -> [w58]
    tunnel: w29 -> [w57]
    tunnel: w25 -> [w54]
    tunnel: w12 -> [w53]
    tunnel: w11 -> [w52]
    tunnel: w9 -> [w50]
    tunnel: w1 -> [w49]
    tunnel: w7 -> [w48]
    tunnel: "Configure (False)" -> [w47]
    tunnel: "TEMPERATURE POINT" -> [w46]
    tunnel: "INITIAL temperature" -> [w44]
    tunnel: "TEMPERATURE STABLE TIME" -> [w43]
    tunnel: w1 -> [w42]
    tunnel: "TEMPERATURE SPACE" -> [w41]
    tunnel: w1 -> [w39]
    frame #0 {
      n3 = call "kethley_INI.vi"("Function (0: Volts) in"=w35, "Source Compaliance"=w37, "VISA Refnum in"=w38) -> ("VISA resource name out"=w36:refnum<visa-resource-name>)  [unwired: 8 in]
    }
    frame #1 {
      n4 = Multiply(x="loop #", y=w46) -> (x*y=w45:i32)
      n5 = stacked-sequence {
        tunnel: "LOCKIN address" -> [_ w82 w137]
        tunnel: w58 -> [_ _ w138]
        tunnel: w57 -> [_ _ w139]
        tunnel: "GATE High Value" -> [_ _ w135]
        tunnel: "GATE Low Value (default 0)" -> [_ _ w136]
        tunnel: w54 -> [_ _ w134]
        tunnel: w45 -> [_ _ w133]
        tunnel: w53 -> [_ _ w131]
        tunnel: w52 -> [_ _ w132]
        tunnel: "lockin-NL" -> [_ w79 w130]
        tunnel: w50 -> [w63 _ w125]
        tunnel: w49 -> [w62 _ _]
        tunnel: w48 -> [w61 _ _]
        tunnel: w47 -> [w60 _ _]
        tunnel: w44 -> [_ _ w127]
        tunnel: w43 -> [_ _ w129]
        tunnel: w42 -> [_ _ w128]
        tunnel: w41 -> [_ _ w126]
        tunnel: "loop #" -> [_ _ w124]
        tunnel: w39 -> [_ _ w123]
        frame #0 {
          n6 = case shown="True" w60 {
            tunnel: [w64 w67] -> _
            tunnel: [w66 w70] -> _
            tunnel: w62 -> [w65 w69]
            tunnel: [w65 w68] -> _
            tunnel: w61 -> [w66 _]
            tunnel: w63 -> [w64 w67]
            frame False {
              # "Do not configure Loop and Setpoint."
            }
            frame True {
              # "Configure Loop and Setpoint."
              n7 = call "Configure Control Parameters.vi"("VISA resource name"=w69, "Manual Output (0.000 %)"="Manual Output (0.000)", "Heater Range (0: Off)"="Heater Range (0: Off)", "Loop (0: 1)"=w67, "Gain (P) (0.0)"="Gain (P) (0.0)", "Reset (I) (0.0)"="Reset (I) (0.0)", "Rate (D) (0)"="Rate (D) (0)") -> ("VISA resource name out"=w68:refnum<visa-resource-name>, "error out"=w76:errorcluster)  [unwired: 7 in]
              n8 = stacked-sequence {
                tunnel: w76 -> [w77]
                tunnel: [w77] -> w70
                frame #0 {
                  # "Wait for loop to \nconfigure."
                  n9 = Wait (ms)(milliseconds to wait=u32 1000) -> ()  [unwired: 1 out]
                }
              }
            }
          }
        }
        frame #1 {
          n10 = call "Abort.vi"("VISA resource name"=w82) -> ("error out"=w80:errorcluster, "VISA resource name out"=w81:refnum<visa-resource-name>)  [unwired: 9 in]
          n11 = flat-sequence {
            tunnel: w81 -> [w101]
            tunnel: [w86] -> w83
            tunnel: w80 -> [w85]
            tunnel: w83 -> [_]
            tunnel: w79 -> [w105]
            frame #0 {
              n12 = call "Configure Trigger.vi"("error in (no error)"=w85, "Trigger Source (0: Internal)"=0, "VISA resource name"=w101) -> ("error out"=w95:errorcluster, "VISA resource name out"=w96:refnum<visa-resource-name>)  [unwired: 7 in]
              n13 = call "Configure Reference.vi"("VISA resource name"=w96, "Auto Phase (T: Enabled)"="auto phase", "Manual Phase (0 Degree)"="manual phase", "Reference Source (1: Internal)"=1, "Sine Output Amplitude (1 V)"="Sine Output Amplitude (1 V) 2", "Detection Harmonic Number (1)"="harm#2", "error in (no error)"=w95, "Internal Reference Frequency (1000 Hz)"="frequency") -> ("VISA resource name out"=w93:refnum<visa-resource-name>, "error out"=w88:errorcluster)  [unwired: 6 in]
              n14 = call "Configure Acquisition.vi"("Continuous Storage (T: Enable)"=FALSE, "error in (no error)"=w88, "VISA resource name"=w93) -> ("error out"=w87:errorcluster, "VISA resource name out"=w91:refnum<visa-resource-name>)  [unwired: 7 in]
              n15 = call "Configure Input Signal.vi"("error in (no error)"=w87, "Input Connection (0: Single-Ended Voltage)"="Input Connection (0: Single-Ended Voltage)", "VISA resource name"=w91) -> ("error out"=w86:errorcluster)  [unwired: 7 in, 1 out]
            }
            frame #1 {
              n16 = Multiply(x="SD stabilization(S) 2", y=1000) -> (x*y=w104:dbl)
              n17 = Wait (ms)(milliseconds to wait=w104) -> ()  [unwired: 1 out]
            }
            frame #2 {
              n18 = call "Abort.vi"("VISA resource name"=w105) -> ("error out"=w106:errorcluster, "VISA resource name out"=w107:refnum<visa-resource-name>)  [unwired: 9 in]
              n19 = call "Configure Trigger.vi"("error in (no error)"=w106, "Trigger Source (0: Internal)"="TRIGGER (1:EXTERNAL)", "VISA resource name"=w107) -> ("error out"=w117:errorcluster, "VISA resource name out"=w118:refnum<visa-resource-name>)  [unwired: 7 in]
              n20 = call "Configure Reference.vi"("VISA resource name"=w118, "Auto Phase (T: Enabled)"="auto phase 2", "Manual Phase (0 Degree)"="manual phase 2", "Reference Source (1: Internal)"="REFERENCE(0:EXTERNAL)", "Sine Output Amplitude (1 V)"="Sine Output Amplitude (1 V) 3", "Detection Harmonic Number (1)"="harm#2 2", "error in (no error)"=w117, "Internal Reference Frequency (1000 Hz)"="frequency 2") -> ("VISA resource name out"=w115:refnum<visa-resource-name>, "error out"=w110:errorcluster)  [unwired: 6 in]
              n21 = call "Configure Acquisition.vi"("Continuous Storage (T: Enable)"=FALSE, "error in (no error)"=w110, "VISA resource name"=w115) -> ("error out"=w109:errorcluster, "VISA resource name out"=w113:refnum<visa-resource-name>)  [unwired: 7 in]
              n22 = call "Configure Input Signal.vi"("error in (no error)"=w109, "Input Connection (0: Single-Ended Voltage)"="Input Connection (0: Single-Ended Voltage)  2", "VISA resource name"=w113) -> ()  [unwired: 7 in, 2 out]
            }
          }
        }
        frame #2 {
          n23 = for {
            N: w133 -> [_]
            tunnel: w139 -> [w174]
            tunnel: w138 -> [w173]
            tunnel: w137 -> [w172]
            tunnel: w136 -> [w171]
            tunnel: w135 -> [w170]
            tunnel: w134 -> [w169]
            shift-right: [w168] -> _
            shift-left: _ -> [w167]
            shift-right: [w166] -> _
            shift-left: _ -> [w164]
            shift-right: [w165] -> _
            shift-left: _ -> [w163]
            tunnel: w132 -> [w161]
            tunnel: w131 -> [w160]
            shift-right: [w159] -> _
            shift-left: _ -> [w158]
            shift-right: [w157] -> _
            shift-left: _ -> [w156]
            tunnel: w130 -> [w155]
            shift-right: [w154] -> _
            shift-left: _ -> [w153]
            shift-right: [w152] -> _
            shift-left: _ -> [w151]
            shift-right: [w150] -> _
            shift-left: _ -> [w149]
            tunnel: w129 -> [w148]
            tunnel: w128 -> [w147]
            tunnel: w127 -> [w144]
            tunnel: w126 -> [w143]
            tunnel: w125 -> [w142]
            tunnel: w124 -> [w141]
            tunnel: w123 -> [w140]
            i -> [w146]
            n24 = Add(x=1, y=w146) -> (x+y=w145:i32)
            "loop run" <- w145
            n25 = stacked-sequence {
              tunnel: w174 -> [_ w251]
              tunnel: w173 -> [_ w250]
              tunnel: w172 -> [_ w249]
              tunnel: w171 -> [_ w243]
              tunnel: w170 -> [_ w242]
              tunnel: w169 -> [_ w241]
              tunnel: [_ w237] -> w168
              tunnel: w167 -> [_ w236]
              tunnel: [_ w235] -> w166
              tunnel: [_ w234] -> w165
              tunnel: w164 -> [_ w233]
              tunnel: w163 -> [_ w232]
              tunnel: w161 -> [_ w231]
              tunnel: w160 -> [_ w230]
              tunnel: [_ w229] -> w159
              tunnel: w158 -> [_ w228]
              tunnel: [_ w227] -> w157
              tunnel: w156 -> [_ w226]
              tunnel: w155 -> [_ w225]
              tunnel: [_ w224] -> w154
              tunnel: w153 -> [_ w223]
              tunnel: [_ w222] -> w152
              tunnel: w151 -> [_ w221]
              tunnel: [_ w220] -> w150
              tunnel: w149 -> [_ w219]
              tunnel: w148 -> [w185 _]
              tunnel: w147 -> [w184 _]
              tunnel: w145 -> [w181 _]
              tunnel: w144 -> [w180 _]
              tunnel: w143 -> [w178 _]
              tunnel: w142 -> [w177 _]
              tunnel: w141 -> [w176 _]
              tunnel: w140 -> [_ w218]
              frame #0 {
                n26 = Quotient & Remainder(x=w181, y=w176) -> (x-y*floor(x/y)=w183:i32, floor(x/y)=w179:i32)
                n27 = Equal?(x=w183, y=1) -> (x = y?=w175:bool)
                n28 = case shown="True" w175 {
                  tunnel: w185 -> [_ w196]
                  tunnel: w184 -> [_ w194]
                  tunnel: w180 -> [_ w191]
                  tunnel: w179 -> [_ w190]
                  tunnel: w178 -> [_ w189]
                  tunnel: w177 -> [_ w187]
                  frame False {
                  }
                  frame True {
                    # "Wait after configuration\nto read data."
                    n29 = Multiply(x=w189, y=w190) -> (x*y=w188:i32)
                    n30 = Add(x=w191, y=w188) -> (x+y=w186:i32)
                    "TEMPERATURE SET" <- w186
                    n31 = call "Configure Setpoint.vi"("VISA resource name"=w194, "Loop (0: 1)"=w187, "Setpoint (0.0000)"=w186) -> ("VISA resource name out"=w193:refnum<visa-resource-name>, "error out"=w192:errorcluster)  [unwired: 11 in]
                    n32 = Wait (ms)(milliseconds to wait=1000) -> ()  [unwired: 1 out]
                    n33 = while {
                      tunnel: w193 -> [w210]
                      tunnel: w192 -> [w209]
                      tunnel: [w203] -> w195
                      tunnel: w186 -> [w202]
                      stop <- w205 stop-if-true
                      # "Get sensor and heater\noutput data."
                      n34 = call "Read Sensor.vi"("VISA resource name"=w210, "Input (0: A)"="Input (0: A) 2", "error in (no error)"=w209) -> ("VISA resource name out"=w215:refnum<visa-resource-name>, "Kelvin Reading"=w208:dbl, "error out"=w214:errorcluster)  [unwired: 8 in, 2 out]
                      "Kelvin Reading 2" <- w208
                      n35 = call "Read Heater Output.vi"("VISA resource name"=w215, "error in (no error)"=w214) -> ("VISA resource name out"=w212:refnum<visa-resource-name>, "Loop 1\nHeater Output"=→"Loop 1\nHeater Output 2":dbl, "error out"=w213:errorcluster)  [unwired: 11 in]
                      n36 = Subtract(x=w208, y=w202) -> (x-y=w207:dbl)
                      n37 = Absolute Value(x=w207) -> (abs(x)=w206:dbl)
                      n38 = call "Close.vi"("VISA resource name"=w212, "error in (no error)"=w213) -> ("error out"=w217:errorcluster)  [unwired: 13 in]
                      n39 = call <vilib>:"Simple Error Handler.vi"("error in (no error)"=w217) -> ("error out"=w203:errorcluster)  [unwired: 4 in, 4 out]
                      n40 = Less?(x=w206, y=0.1) -> (x < y?=w205:bool)
                    }
                    n41 = stacked-sequence {
                      tunnel: w195 -> [w201]
                      tunnel: [w201] -> _
                      tunnel: w196 -> [w198]
                      frame #0 {
                        # "Wait after configuration\nto read data."
                        n42 = Multiply(x=w198, y=60000) -> (x*y=w199:i32)
                        n43 = Wait (ms)(milliseconds to wait=w199) -> ()  [unwired: 1 out]
                      }
                    }
                  }
                }
              }
              frame #1 {
                n44 = Subtract(x=w242, y=w243) -> (x-y=w245:dbl)
                n45 = Divide(x="GATE STEP(mv)", y=1000) -> (x/y=w244:dbl)
                n46 = Divide(x=w245, y=w244) -> (x/y=w240:dbl)
                n47 = Multiply(x=4, y=w240) -> (x*y=w239:dbl)
                n48 = Increment(x=w239) -> (x+1=w238:dbl)
                n49 = for {
                  N: w238 -> [_]
                  tunnel: w251 -> [w297]
                  tunnel: w250 -> [w296]
                  tunnel: w249 -> [w295]
                  tunnel: w244 -> [w286]
                  shift-right: [w294] -> w237
                  shift-left: w236 -> [w293]
                  shift-right: [w290] -> w234
                  shift-left: w232 -> [w292]
                  shift-right: [w289] -> w235
                  shift-left: w233 -> [w291]
                  tunnel: w240 -> [w284]
                  tunnel: w243 -> [w287]
                  tunnel: w242 -> [w285]
                  tunnel: w241 -> [w279]
                  tunnel: w231 -> [w272]
                  tunnel: w230 -> [w271]
                  shift-right: [w270] -> w229
                  shift-left: w228 -> [w269]
                  shift-right: [w266] -> w227
                  shift-left: w226 -> [w265]
                  tunnel: w225 -> [w263]
                  shift-right: [w261] -> w224
                  shift-left: w223 -> [w260]
                  shift-right: [w259] -> w222
                  shift-left: w221 -> [w258]
                  shift-right: [w255] -> w220
                  shift-left: w219 -> [w256]
                  tunnel: w218 -> [w252]
                  i -> [w283]
                  n50 = Divide(x="bottom gate thickness", y="top gate thickness") -> (x/y=w277:dbl)
                  n51 = Less Or Equal?(x=w283, y=w284) -> (x <= y?=w288:bool)
                  n52 = case shown="False" w288 {
                    tunnel: w287 -> [_ w349]
                    tunnel: w283 -> [w329 w348]
                    tunnel: w286 -> [w328 w347]
                    tunnel: [w326 w345] -> w267
                    tunnel: w285 -> [w327 _]
                    tunnel: w284 -> [w322 _]
                    tunnel: w283 -> [w325 _]
                    frame False {
                      n53 = Multiply(x=w322, y=3) -> (x*y=w321:dbl)
                      n54 = Less Or Equal?(x=w325, y=w321) -> (x <= y?=w323:bool)
                      n55 = case shown="False" w323 {
                        tunnel: w329 -> [w337 w344]
                        tunnel: w328 -> [w335 w342]
                        tunnel: w327 -> [w331 w340]
                        tunnel: [w333 w339] -> w326
                        tunnel: w322 -> [_ w338]
                        tunnel: w321 -> [w330 _]
                        frame False {
                          n56 = Negate(x=w331) -> (-x=w332:dbl)
                          n57 = Subtract(x=w337, y=w330) -> (x-y=w336:dbl)
                          n58 = Multiply(x=w335, y=w336) -> (x*y=w334:dbl)
                          n59 = Add(x=w332, y=w334) -> (x+y=w333:dbl)
                        }
                        frame True {
                          n60 = Subtract(x=w344, y=w338) -> (x-y=w343:dbl)
                          n61 = Multiply(x=w342, y=w343) -> (x*y=w341:dbl)
                          n62 = Subtract(x=w340, y=w341) -> (x-y=w339:dbl)
                        }
                      }
                    }
                    frame True {
                      n63 = Multiply(x=w347, y=w348) -> (x*y=w346:dbl)
                      n64 = Add(x=w349, y=w346) -> (x+y=w345:dbl)
                    }
                  }
                  n65 = case shown="True" "pure field (T)/pure doping (F)" {
                    tunnel: w277 -> [w301 w307]
                    tunnel: [w298 w305] -> w273
                    tunnel: w267 -> [w299 w304]
                    frame False {
                      n66 = Multiply(x=w301, y=1) -> (x*y=w300:dbl)
                      n67 = Divide(x=w299, y=w300) -> (x/y=w298:dbl)
                    }
                    frame True {
                      n68 = Multiply(x=w307, y=-1) -> (x*y=w303:dbl)
                      n69 = Divide(x=w304, y=w303) -> (x/y=w305:dbl)
                    }
                  }
                  n70 = stacked-sequence {
                    tunnel: w297 -> [w356 _ _ _ _ _]
                    tunnel: w296 -> [w355 _ w380 _ _ _]
                    tunnel: w295 -> [_ _ _ w415 _ _]
                    tunnel: w267 -> [w354 _ _ w413 w457 _]
                    tunnel: [_ _ w378 _ _ _] -> w294
                    tunnel: w293 -> [_ _ w379 _ _ _]
                    tunnel: w292 -> [_ _ _ w419 _ _]
                    tunnel: w291 -> [_ _ _ w416 _ _]
                    tunnel: [_ _ _ w418 _ _] -> w290
                    tunnel: [_ _ _ w417 _ _] -> w289
                    tunnel: [_ _ _ w414 _ _] -> w282
                    tunnel: [_ _ _ w413 _ _] -> w281
                    tunnel: [_ _ w376 _ _ _] -> w280
                    tunnel: w273 -> [w351 _ _ _ _ _]
                    tunnel: w272 -> [_ _ w368 _ _ _]
                    tunnel: w271 -> [w350 _ w367 _ _ _]
                    tunnel: [_ _ w366 _ _ _] -> w270
                    tunnel: w269 -> [_ _ w365 _ _ _]
                    tunnel: [_ _ w364 _ _ _] -> w268
                    tunnel: w267 -> [_ _ _ _ _ _]
                    tunnel: [_ _ _ w406 _ _] -> w266
                    tunnel: w265 -> [_ _ _ w405 _ _]
                    tunnel: [_ _ _ w404 _ _] -> w264
                    tunnel: w263 -> [_ _ _ _ w458 _]
                    tunnel: [_ _ _ _ w456 _] -> w262
                    tunnel: [_ _ _ _ w455 _] -> w261
                    tunnel: w260 -> [_ _ _ _ w454 _]
                    tunnel: [_ _ _ _ w453 _] -> w259
                    tunnel: w258 -> [_ _ _ _ w452 _]
                    tunnel: [_ _ _ _ w451 _] -> w257
                    tunnel: w256 -> [_ _ _ _ w450 _]
                    tunnel: [_ _ _ _ w449 _] -> w255
                    tunnel: [_ _ _ w403 _ _] -> w254
                    tunnel: [_ _ _ _ _ w495] -> w253
                    tunnel: w252 -> [_ _ _ _ _ w494]
                    frame #0 {
                      w358 = "VOLT\nCURR"  # Source Function
                      w359 = ":SOUR:%s %g;"  # Manual Range
                      n71 = Pick Line(multi-line string=w358, line index=w356) -> (output string=w357:string)  [unwired: 1 out]
                      n72 = Format Into String(format string=w359, w357, w354) -> (resulting string=w360:string)  [unwired: 2 in, 1 out]
                      n73 = VISA Write(VISA resource name=w355, write buffer=w360) -> ()  [unwired: 1 in, 3 out]
                      n74 = call <instrlib>:"Configure Output.vi"("Source Mode  (0: Voltage)"="Source Mode  (0: Voltage)", "Compliance  Level (0.1)"="Compliance  Level (1uA)", "Output Level (0)"=w351, "VISA resource name"=w350) -> ()  [unwired: 6 in, 2 out]
                      "gate voltage" <- w354
                      "top gate voltage" <- w351
                    }
                    frame #1 {
                      n75 = Multiply(x="LOCKIN-WAIT", y=1000) -> (x*y=w363:dbl)
                      n76 = Wait (ms)(milliseconds to wait=w363) -> ()  [unwired: 1 out]
                    }
                    frame #2 {
                      w373 = u16 0 items=["Fixed", "Sweep", "List"]  # Output Mode (0: Fixed)
                      w391 = "defbuffer1" ("Buffer Name (defbuffer1) 2")
                      (unwired) "defbuffer1" ("t")
                      w389 = "\""
                      w386 = ":READ?"  # Read Measurement
                      w395 = u32 10000  # Bytes
                      # "NOTE :\nBuffer Elements :\nDATE\nFORM\nFRAC\nREAD\nREL\nSEC\nSOUR\nSOURFORM\nSOURSTAT\nSOURUNIT\nSTAT\nTIME\nTsT\nUNIT"
                      # ":READ? \"<BufferName>\", <Buffer Element>"
                      # "SCPI 2450"
                      n77 = call <instrlib>:"Enable Output.vi"("error in (no error)"=w368, "Enable Output (T: Enable)"=TRUE, "VISA resource name"=w367) -> ("VISA resource name out"=w369:refnum<visa-resource-name>)  [unwired: 7 in, 1 out]
                      n78 = Equal?(x="", y=w391) -> (x = y?=w392:bool)
                      n79 = call-poly <instrlib>:"Read.vi"("VISA resource name"=w369, "Sample Count (1)"=u32 2 ("Number of Samples"), "Timeout (10000 ms)"=1000, "Output Mode (0: Fixed)"=w373) -> ("Voltage"=w371:sgl[], "Current"=w372:sgl[])  [unwired: 5 in, 5 out]
                      n80 = Select(t="defbuffer1", s=w392, f=w391) -> (s? t:f=w388:string)
                      n81 = call <vilib>:"Std Deviation and Variance.vi"("X"=w371) -> ()  [unwired: 1 in, 3 out]
                      n82 = call <vilib>:"Space Constant.vi"() -> ("String"=w387:string)
                      n83 = call <vilib>:"Std Deviation and Variance.vi"("X"=w372) -> ("mean"=w364:dbl)  [unwired: 1 in, 2 out]
                      "top gate leaking" <- w364
                      n84 = Concatenate Strings(w386, w387, w389, w388, w389, ", " ("string"), "READ" ("Buffer Elements 2")) -> (w402:string)
                      n85 = VISA Write(VISA resource name=w380, write buffer=w402) -> (VISA resource name out=w394:refnum<visa-resource-name>, error out=w401:errorcluster)  [unwired: 1 in, 1 out]
                      n86 = property class="Instr"(reference=w394, error in=w401, "General Settings:Timeout Value"=10000 ("Timeout (10000 ms) 2")) -> (reference out=w400:refnum<visa-resource-name>, error out=w399:errorcluster, "General Settings:Timeout Value"=w396:u32)
                      n87 = VISA Read(VISA resource name=w400, byte count=w395, error in (no error)=w399) -> (VISA resource name out=w398:refnum<visa-resource-name>, read buffer=w377:string, error out=w397:errorcluster)  [unwired: 1 out]
                      "gate leaking" <- w377
                      n88 = property class="Instr"(reference=w398, error in=w397, "General Settings:Timeout Value"=w396) -> (reference out=w384:refnum<visa-resource-name>, error out=w383:errorcluster)
                      n89 = Fract/Exp String To Number(string=w377) -> (number=w376:dbl)  [unwired: 3 in, 1 out]
                      n90 = call "Error Query.vi"("error in (no error)"=w383, "VISA resource name"=w384) -> ()  [unwired: 10 out]
                      n91 = Build Array (concatenate)(w376, w379) -> (w378:dbl[])
                      n92 = Build Array (concatenate)(w364, w365) -> (w366:dbl[])
                    }
                    frame #3 {
                      n93 = flat-sequence {
                        tunnel: w419 -> [w429]
                        tunnel: w416 -> [w426]
                        tunnel: w415 -> [w425]
                        tunnel: w413 -> [w423]
                        tunnel: [w421] -> _
                        tunnel: [w422] -> _
                        tunnel: [w428] -> w412
                        tunnel: [w427] -> w411
                        tunnel: [w424] -> w410
                        tunnel: [w422] -> w409
                        tunnel: [w421] -> w408
                        tunnel: ["Clear Plot"] -> w407
                        tunnel: [w447] -> w414
                        tunnel: [w441] -> w417
                        tunnel: [w448] -> w418
                        tunnel: w412 -> [w448]
                        tunnel: w411 -> [w441]
                        tunnel: w410 -> [w447]
                        tunnel: w409 -> [w445]
                        tunnel: w408 -> [w444]
                        tunnel: w407 -> [w442]
                        tunnel: [w439] -> w406
                        tunnel: w405 -> [w438]
                        tunnel: [w436] -> w404
                        frame #0 {
                          n94 = Format Into String(0) -> (error out=w435:errorcluster)  [unwired: 3 in, 1 out]
                          n95 = call "Read (1 Parameter).vi"("error in (no error)"=w435, "Parameter (1: X)"="Parameter (1: X)", "VISA resource name"=w425) -> ("error out"=w422:errorcluster, "Measurement"=w424:dbl, "VISA resource name out"=w421:refnum<visa-resource-name>)  [unwired: 6 in]
                          "para1 Measurement" <- w424
                          n96 = Build Array(w424) -> (w432:dbl[])
                          n97 = Select(t=w432, s="Clear Plot", f=w429) -> (s? t:f=w433:dbl[])
                          n98 = Build Array (concatenate)(w423, w426) -> (w427:dbl[])
                          n99 = Build Array (concatenate)(w424, w433) -> (w428:dbl[])
                          n100 = Bundle(w427, w428) -> (→"XY Graph":cluster{dbl[], dbl[]})  [unwired: 1 in]
                        }
                        frame #1 {
                          n101 = call "Read (1 Parameter).vi"("error in (no error)"=w445, "Parameter (1: X)"="Parameter2 (1: X)", "VISA resource name"=w444) -> ("Measurement"=w436:dbl)  [unwired: 6 in, 2 out]
                          "para2 Measurement" <- w436
                          n102 = Build Array(w436) -> (w443:dbl[])
                          n103 = Select(t=w443, s=w442, f=w438) -> (s? t:f=w440:dbl[])
                          n104 = Build Array (concatenate)(w436, w440) -> (w439:dbl[])
                          n105 = Bundle(w441, w439) -> (→"XY Graph 2":cluster{dbl[], dbl[]})  [unwired: 1 in]
                        }
                      }
                      n106 = property on="TEMPERATURE SET" class="DigNum (strict)"() -> ("Value"=w403:i32)  [unwired: 2 in, 2 out]
                    }
                    frame #4 {
                      n107 = flat-sequence {
                        tunnel: w458 -> [w473]
                        tunnel: w457 -> [w471]
                        tunnel: [w469] -> _
                        tunnel: [w470] -> _
                        tunnel: [w475] -> w464
                        tunnel: [w474] -> w463
                        tunnel: [w472] -> w462
                        tunnel: [w470] -> w461
                        tunnel: [w469] -> w460
                        tunnel: ["Clear Plot 2"] -> w459
                        tunnel: w452 -> [w467]
                        tunnel: w450 -> [w465]
                        tunnel: [w492] -> w451
                        tunnel: [w486] -> w449
                        tunnel: [w493] -> w453
                        tunnel: w464 -> [w493]
                        tunnel: w463 -> [w486]
                        tunnel: w462 -> [w492]
                        tunnel: w461 -> [w490]
                        tunnel: w460 -> [w489]
                        tunnel: w459 -> [w487]
                        tunnel: [w484] -> w455
                        tunnel: [w482] -> _
                        tunnel: [w482] -> w456
                        tunnel: w454 -> [w481]
                        frame #0 {
                          n108 = Format Into String(0) -> (error out=w480:errorcluster)  [unwired: 3 in, 1 out]
                          n109 = call "Read (1 Parameter).vi"("error in (no error)"=w480, "Parameter (1: X)"="Parameter (1: X) 2", "VISA resource name"=w473) -> ("error out"=w470:errorcluster, "Measurement"=w472:dbl, "VISA resource name out"=w469:refnum<visa-resource-name>)  [unwired: 6 in]
                          "R Measurement 2" <- w472
                          n110 = Build Array(w472) -> (w478:dbl[])
                          n111 = Select(t=w478, s="Clear Plot 2", f=w467) -> (s? t:f=w466:dbl[])
                          n112 = Build Array (concatenate)(w471, w465) -> (w474:dbl[])
                          n113 = Build Array (concatenate)(w472, w466) -> (w475:dbl[])
                          n114 = Bundle(w474, w475) -> (→"LOVK2-r":cluster{dbl[], dbl[]})  [unwired: 1 in]
                        }
                        frame #1 {
                          n115 = call "Read (1 Parameter).vi"("error in (no error)"=w490, "Parameter (1: X)"="Parameter2 (1: X)  2", "VISA resource name"=w489) -> ("Measurement"=w482:dbl)  [unwired: 6 in, 2 out]
                          "PHASE" <- w482
                          n116 = Build Array(w482) -> (w488:dbl[])
                          n117 = Select(t=w488, s=w487, f=w481) -> (s? t:f=w485:dbl[])
                          n118 = Build Array (concatenate)(w482, w485) -> (w484:dbl[])
                          n119 = Bundle(w486, w484) -> (→"LOCKIN2\n-THETA":cluster{dbl[], dbl[]})  [unwired: 1 in]
                        }
                      }
                    }
                    frame #5 {
                      n120 = call "Read Sensor.vi"("VISA resource name"=w494, "Input (0: A)"="Input (0: A) 3") -> ("Kelvin Reading"=w495:dbl)  [unwired: 9 in, 4 out]
                      "Kelvin Reading 3" <- w495
                    }
                  }
                  n121 = case shown="True" "Save data or not" {
                    tunnel: w282 -> [_ w320]
                    tunnel: w281 -> [_ w319]
                    tunnel: w280 -> [_ w318]
                    tunnel: w279 -> [_ w316]
                    tunnel: w268 -> [_ w313]
                    tunnel: w264 -> [_ w312]
                    tunnel: w262 -> [_ w311]
                    tunnel: w257 -> [_ w310]
                    tunnel: w254 -> [_ w309]
                    tunnel: w253 -> [_ w308]
                    frame False {
                    }
                    frame True {
                      n122 = Build Array(w319, w320, w309, w308, w312, w313, w318, w310, w311) -> (w317:dbl[])
                      n123 = call-poly <vilib>:"Write To Spreadsheet File.vi"("format (%.3f)"="%.10f", "append to file? (new file:F)"=TRUE, "1D data"=w317, "file path (dialog if empty)"=w316) -> ()  [unwired: 4 in, 1 out]
                    }
                  }
                }
              }
            }
          }
        }
      }
    }
  }
  n124 = call <instrlib>:"Initialize.vi"("Serial Configuration"="Serial Configuration", "VISA resource name"="top gate address") -> ("error out"=w23:errorcluster, "VISA resource name out"=w24:refnum<visa-resource-name>)  [unwired: 8 in]
  n125 = call <instrlib>:"Configure Measurement.vi"("error in (no error)"=w23, "Enable Auto Range (T:Enable)"=w14, "Function (0: Volts)"=w18, "VISA resource name"=w24) -> ("error out"=w22:errorcluster, "VISA resource name out"=w21:refnum<visa-resource-name>)  [unwired: 6 in]
  n126 = call <instrlib>:"Configure Measurement.vi"("error in (no error)"=w22, "Enable Auto Range (T:Enable)"=w14, "Function (0: Volts)"=w17, "VISA resource name"=w21) -> ("error out"=w15:errorcluster, "VISA resource name out"=w16:refnum<visa-resource-name>)  [unwired: 6 in]
  n127 = call <instrlib>:"Configure Measurement.vi"("error in (no error)"=w15, "Enable Auto Range (T:Enable)"=w14, "Function (0: Volts)"=w13, "VISA resource name"=w16) -> ("error out"=w11:errorcluster, "VISA resource name out"=w12:refnum<visa-resource-name>)  [unwired: 6 in]
  n128 = Concatenate Strings("path (folder + filename)", ".txt") -> (w26:string)
  n129 = String To Path(string=w26) -> (path=w25:path)
